vi "AutoBurn - BCU.vi"() -> ()   [LabVIEW 2013]
uses:
  <vilib>/Utility/config.llb/Write Key (String).vi
  <vilib>/Utility/config.llb/Read Key (String).vi
  <vilib>/Utility/file.llb/Read From Spreadsheet File (string).vi
  Settings/ControlCAN.dll
  <vilib>/Utility/config.llb/NI_LVConfig.lvlib
panel:
  out "?":bool
  in  "波特率 2":T1(ring)=enum."500Kbps"
  in  "错误输入（无错误）":errorcluster
  out "开始下载数据":u32
  out "开始下载数据":bool=TRUE
  out "耗时：":u32
  out "start":u32
  out "update flag":bool=TRUE
  in  "目标板类型":enum16{"BCU/主板", "BMU/从板"}(ring)
  out "Random":u32
  out "CRC16":u16 format="%x"
  out "进入烧录":bool
  out "boot模式应答计数":i32
  out "boot模式应答...成功":bool=TRUE
  out "总行数":i32
  in  "错误输入（无错误） 7":errorcluster caption="错误输入（无错误）"
  out "错误输出 18":errorcluster caption="错误输出"
  out "当前发送行":i32
  in  "错误输入（无错误） 6":errorcluster caption="错误输入（无错误）"
  out "错误输出 17":errorcluster caption="错误输出"
  in  "错误输入（无错误） 5":errorcluster caption="错误输入（无错误）"
  out "错误输出 16":errorcluster caption="错误输出"
  in  "错误输入（无错误） 4":errorcluster caption="错误输入（无错误）"
  out "错误输出 15":errorcluster caption="错误输出"
  in  "错误输入（无错误） 3":errorcluster caption="错误输入（无错误）"
  out "错误输出 14":errorcluster caption="错误输出"
  out "错误输出 13":errorcluster caption="错误输出"
  out "错误输出 12":errorcluster caption="错误输出"
  out "总电压":dbl
  out "Life":dbl
  out "返回类型":u32 format="%x"
  out "Info：":string
  in  "手动进入编程模式 2":bool
  out "T9":bool=TRUE
  out "T8":u8
  out "T7":bool=TRUE
  out "T6":bool=TRUE
  out "T5":bool=TRUE
  out "T4":bool=TRUE
  out "T3":bool=TRUE
  out "T2":bool=TRUE
  out "T1":bool=TRUE
  out "ID":u32 format="%x"
  out "错误输出 3":errorcluster caption="错误输出"
  in  "Monitor":bool
  out "校验":bool
  in  "请选择板号":u16(ring)=1 items=["BMU1"=1, "BMU2"=2, "BMU3"=3, "BMU4"=4, "BMU5"=5, "BMU6"=6, "BMU7"=7, "BMU8"=8, "BMU9"=9, "BMU10"=10, "BMU11"=11, "BMU12"=12, "BMU13"=13, "BMU14"=14, "BMU15"=15, "BMU16"=16, "BMU17"=17, "BMU18"=18, "BMU19"=19, "BMU20"=20]
  in  "手动进入编程模式":bool
  in  "板类型":enum16{"请选择板类型", "主板", "从板", "高压板"}(ring)=enum."主板"
  out "烧录结果":bool=TRUE
  out "擦除完成":bool
  out "进入烧录模式":bool
  out "MD5校验":bool
  out "进度":u8(slide) scale=0.0..100.0
  out "校验码实际值":string
  in  "校验码期望值":string
  in  "应用程序路径":path
  out "连接状态":bool=TRUE
  in  "类型":u32(ring)=4 items=["PCI5121"=1, "PCI9810"=2, "USBCAN1"=3, "USBCAN2"=4, "PCI9820"=5, "CAN232"=6, "PCI5110"=7, "CANLite(mini)"=8, "ISA9620"=9, "ISA5420"=10, "PC104CAN"=11, "CANET"=17, "DNP9810"=13, "USBCAN-E-U"=20, "USBCAN-2E-U"=21]
  in  "CAN路数":u32(ring) items=["0", "1"]
  in  "滤波方式":u8(ring) items=["Dual Filter", "Single Filter"]
  in  "工作方式":u8(ring) items=["Normal", "Listen Only"]
  in  "波特率":T1(ring)=enum."500Kbps"
  in  "设备索引":u32(ring) items=["0", "1", "2", "3", "4", "5", "6", "7", "8", "9", "10", "11", "12", "13", "14", "15", ""]
  in  "开始监控":bool
  out "CAN数据":bool
  out "Monitor_flag":bool
  out "PC端-协议类型 2":enum16{"TCP服务器Server", "TCP客户端Client"}(ring)
  out "通信端口:":u32
  out "CANET地址格式如：192.168.0.178":string
  out "发送数据长度":dbl
  out "发送的数据":i32[](array[numeric])
  in  "设备索引 4":u16(ring) items=["0", "1", "2", "3", "4", "5", "6", "7", "8", "9", "10", "11", "12", "13", "14", "15", ""]
  in  "CAN路数 4":u16(ring) items=["0", "1"]
  in  "设备类型 4":u16(ring)=4 items=["PCI5121"=1, "PCI9810"=2, "USBCAN1"=3, "USBCAN2"=4, "PCI9820"=5, "CAN232"=6, "PCI5110"=7, "CANLite(mini)"=8, "ISA9620"=9, "ISA5420"=10, "PC104CAN"=11, "CANETE"=12, "DNP9810"=13]
  out "Mode":bool
  in  "开始监控 2":bool
  out "大小":i32=426
  out "地址长度 2":u32=4
  out "数据长度 2":u32=64
  out "子字符串 2":string="9B2F9B349B399B3E9B439B499B4F9B559B5B9B619B679B6D9B739B799B7F7C7B"
  out "数据长度":u32=64
  out "地址长度":u32=4
  in  "设定":bool
  out "VCI_CAN_OBJ_T":T2 {"ID" format="%x"}
  out "子数组":string[](array[string])
  in  "从板号":dbl
  out "从板号2":dbl
  in  "读取":bool
  in  "停止 3":bool
  out "TEMP":bool
  out "CAN状态 2":bool
  out "VCI_CAN_OBJ_R":T2={"ID"=0, "TimeStamp"=0, "TimeFlag"=0, "SendType"=1, "RemoteFlag"=0, "ExternFlag"=0, "DataLen"=8, 0, 0, 0, 0, 0, 0, 0, 0, 0, 0, 0}
  in  "停止 2":bool
  out "接收":T2={"ID"=0, "TimeStamp"=61537964, "TimeFlag"=1, "SendType"=250, "RemoteFlag"=0, "ExternFlag"=0, "DataLen"=1, 255, 0, 0, 0, 0, 0, 0, 0, 0, 0, 124} {"ID" min=2 max=104373490 step=1 format="%x"; "TimeStamp" min=1962977793 max=3175728; "TimeFlag" min=1 max=0; "SendType" max=131 step=11; "RemoteFlag" min=52 max=6 step=1; "ExternFlag" max=0; "DataLen" min=1 max=170; "?" min=117 max=48 step=117; "?" min=48 max=0; "?" max=0; "?" min=2 max=0; "?" max=150 step=11; "?" min=52 max=6 step=1; "?" max=0; "?" min=1 max=170; "?" min=120 max=175; "?" max=12; "?" max=0}
  out "收到请求":bool=TRUE
  out "分配":bool
  out "设置中？ 2":bool
  in  "Boar_Type":bool
  out "temp1":bool
  out "设置中？":bool
  in  "总步骤":dbl=21.0
  in  "失败重测次数":dbl=3.0
  out "一键测试":bool
  out "测试结果":bool
  in  "行号":dbl=21.0
  in  "工作方式 2":u8(ring) items=["Normal", "Listen Only"]
  in  "设备类型 2":u16(ring)=4 items=["PCI5121"=1, "PCI9810"=2, "USBCAN1"=3, "USBCAN2"=4, "PCI9820"=5, "CAN232"=6, "PCI5110"=7, "CANLite(mini)"=8, "ISA9620"=9, "ISA5420"=10, "PC104CAN"=11, "CANETE"=12, "DNP9810"=13]
  in  "停止":bool
  out "CAN状态":bool=TRUE
  in  "监控":bool
  # "当前BMU信息"
  # "蓝微新源BMS_CAN应用程序下载器V1.0.7D"
  # "注意：升级完成后系统需要重新上电才能正常运行！"
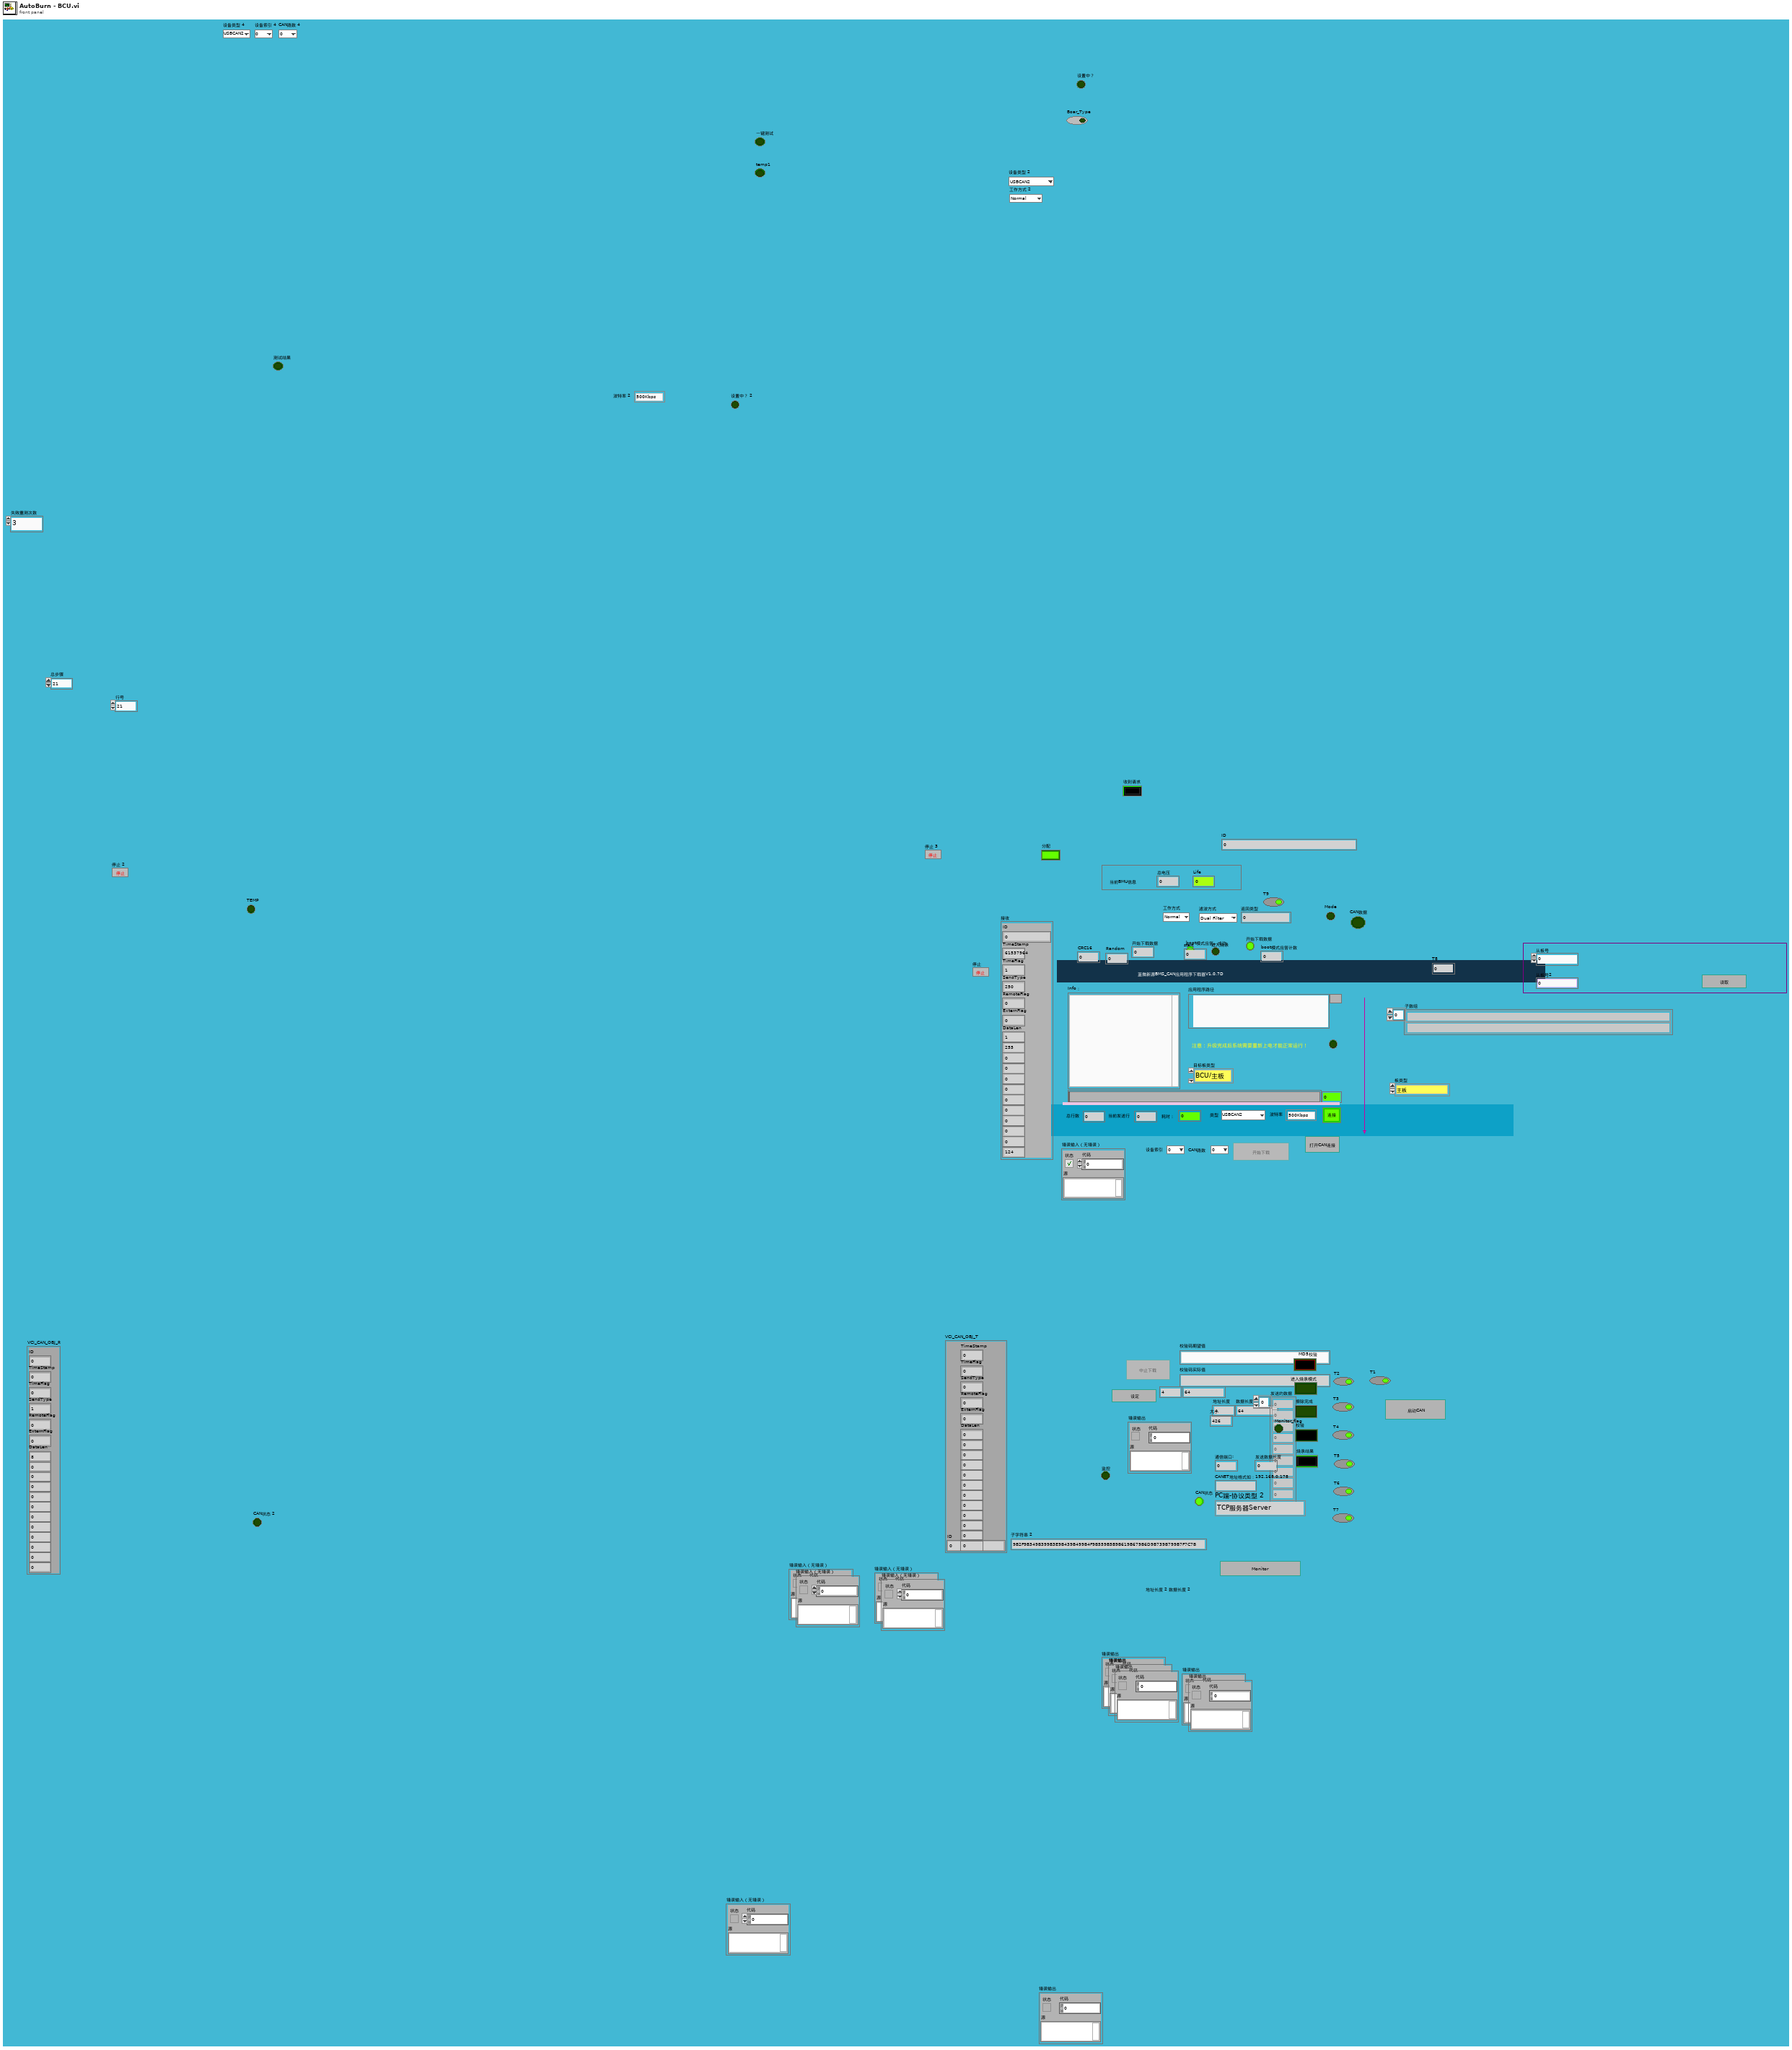
[diagram p1: front panel]
types:
  T1 = enum16{"5Kbps", "10Kbps", "20Kbps", "40Kbps", "50Kbps", "80Kbps", "100Kbps", "125Kbps", "200Kbps", "250Kbps", "400Kbps", "500Kbps", "666Kbps", "800Kbps", "1000Kbps"}
  T2 = cluster{"ID":u32, "TimeStamp":u32, "TimeFlag":u8, "SendType":u8, "RemoteFlag":u8, "ExternFlag":u8, "DataLen":u8, u8, u8, u8, u8, u8, u8, u8, u8, u8, u8, u8}
  T3 = enum8{"Enabled", "Disabled", "Disabled and Grayed Out"}
  T4 = typedef "NI_LVConfig.lvlib/Config Data RefNum.ctl" = refnum<k1>
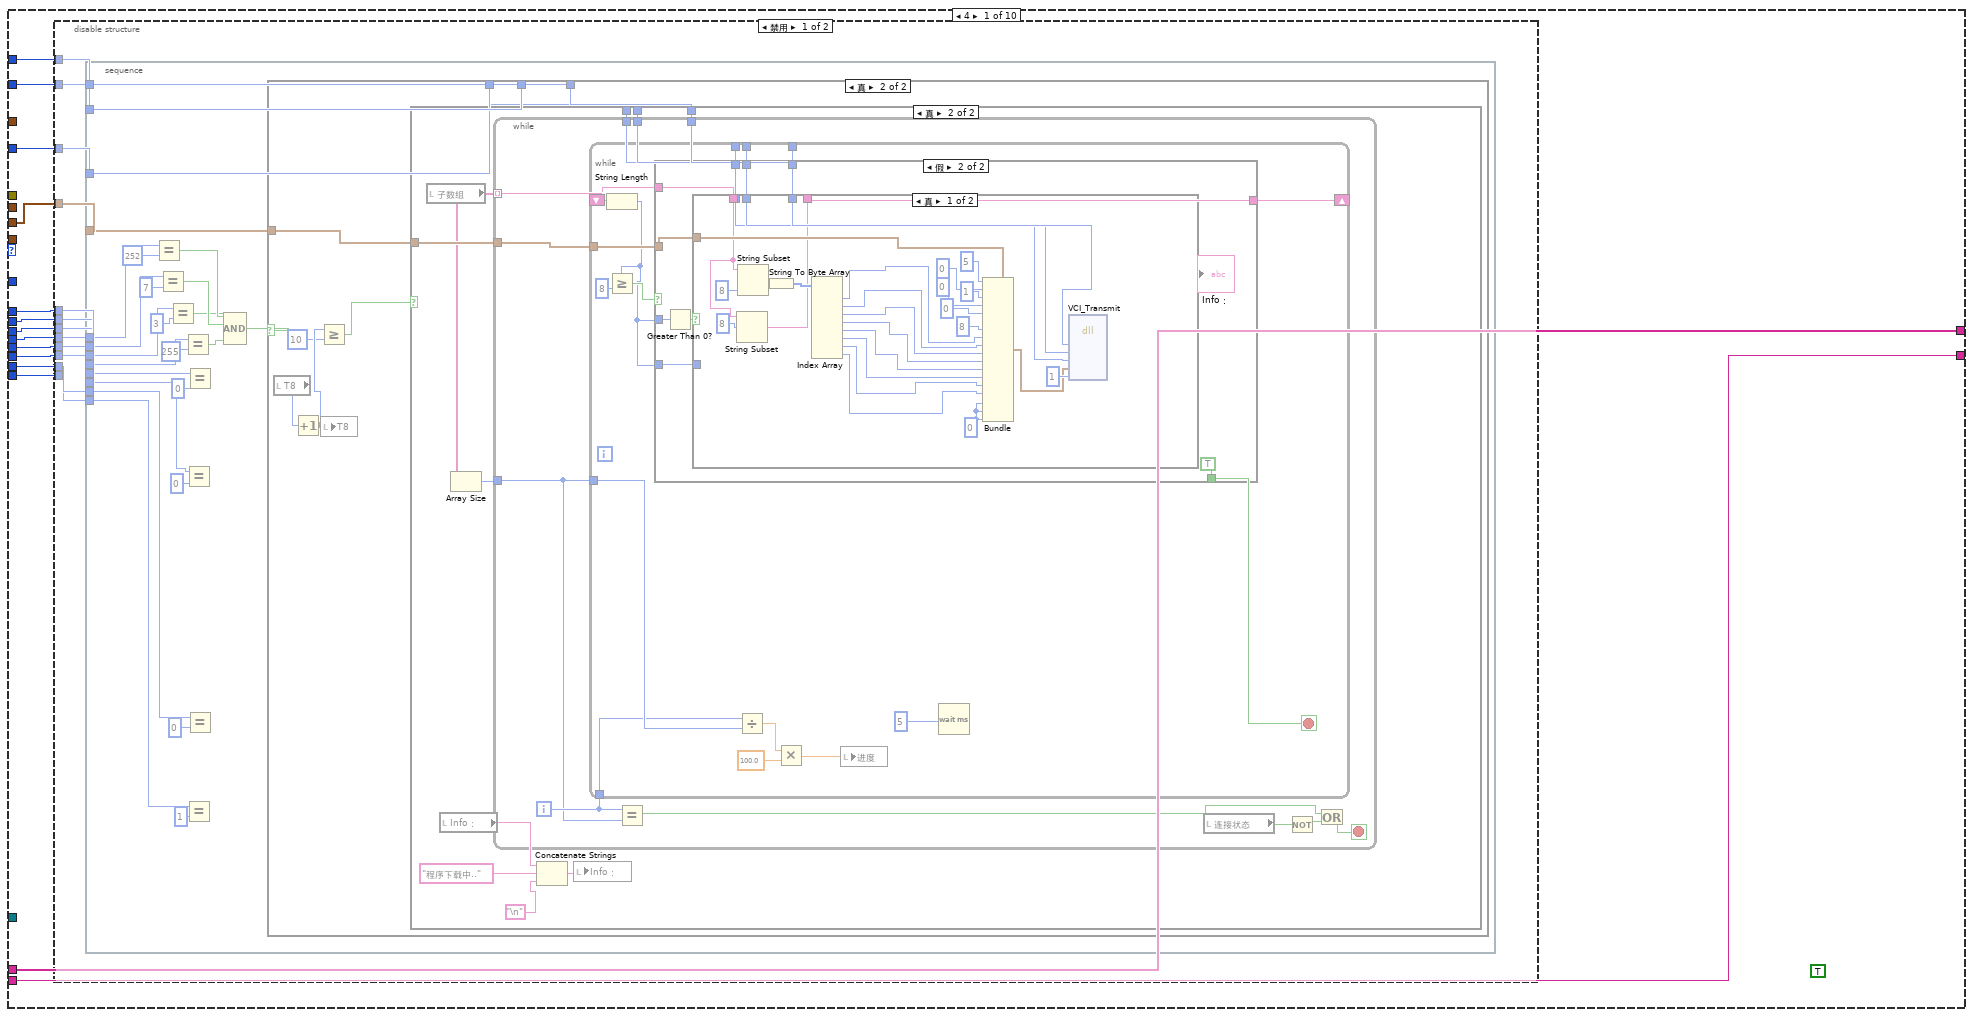
[diagram p3: hidden frame]
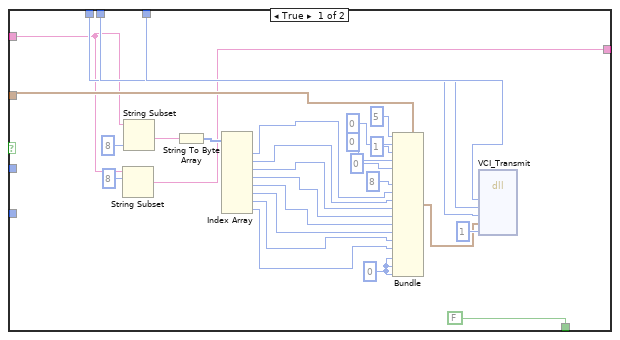
[diagram p6: hidden frame]
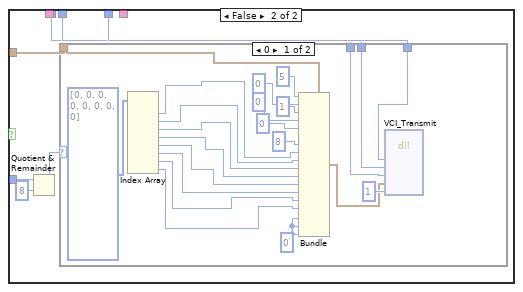
[diagram p7: hidden frame]
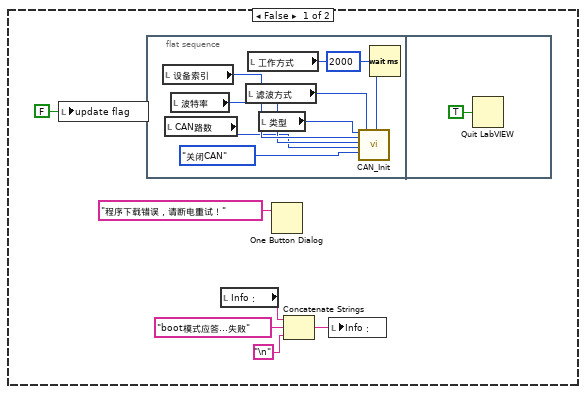
[diagram p10: hidden frame]
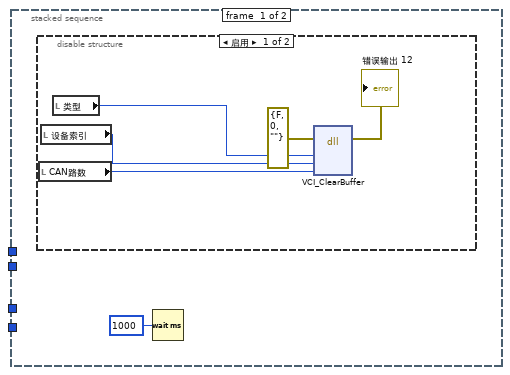
[diagram p11: hidden frame]
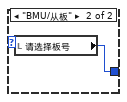
[diagram p13: hidden frame]
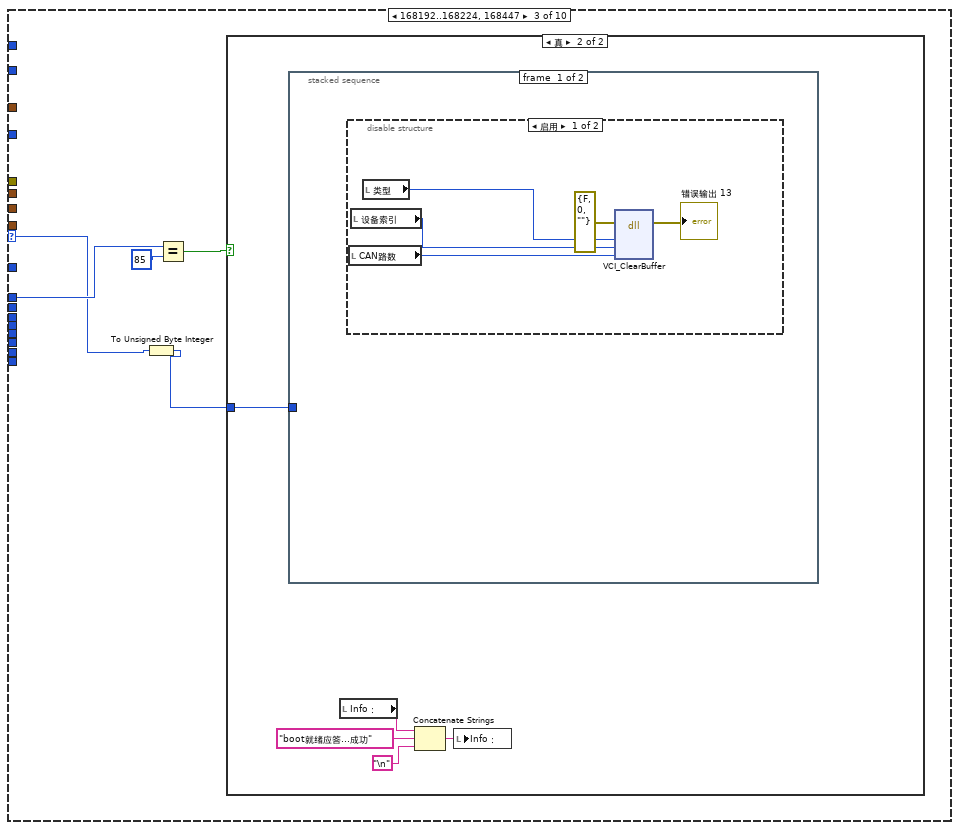
[diagram p14: hidden frame]
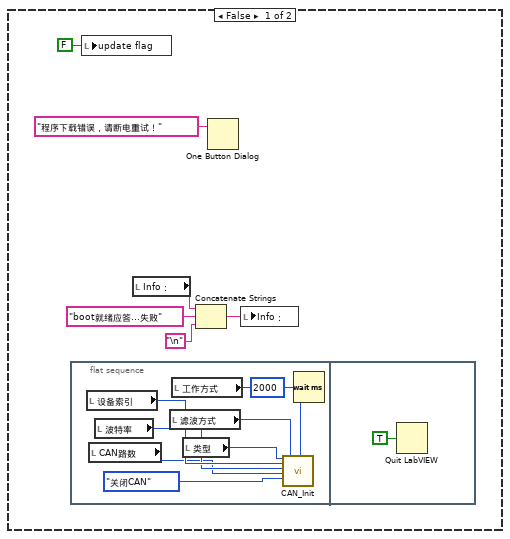
[diagram p15: hidden frame]
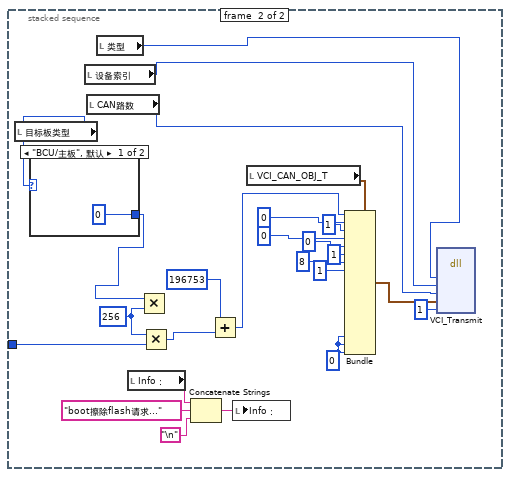
[diagram p17: hidden frame]
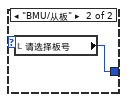
[diagram p18: hidden frame]
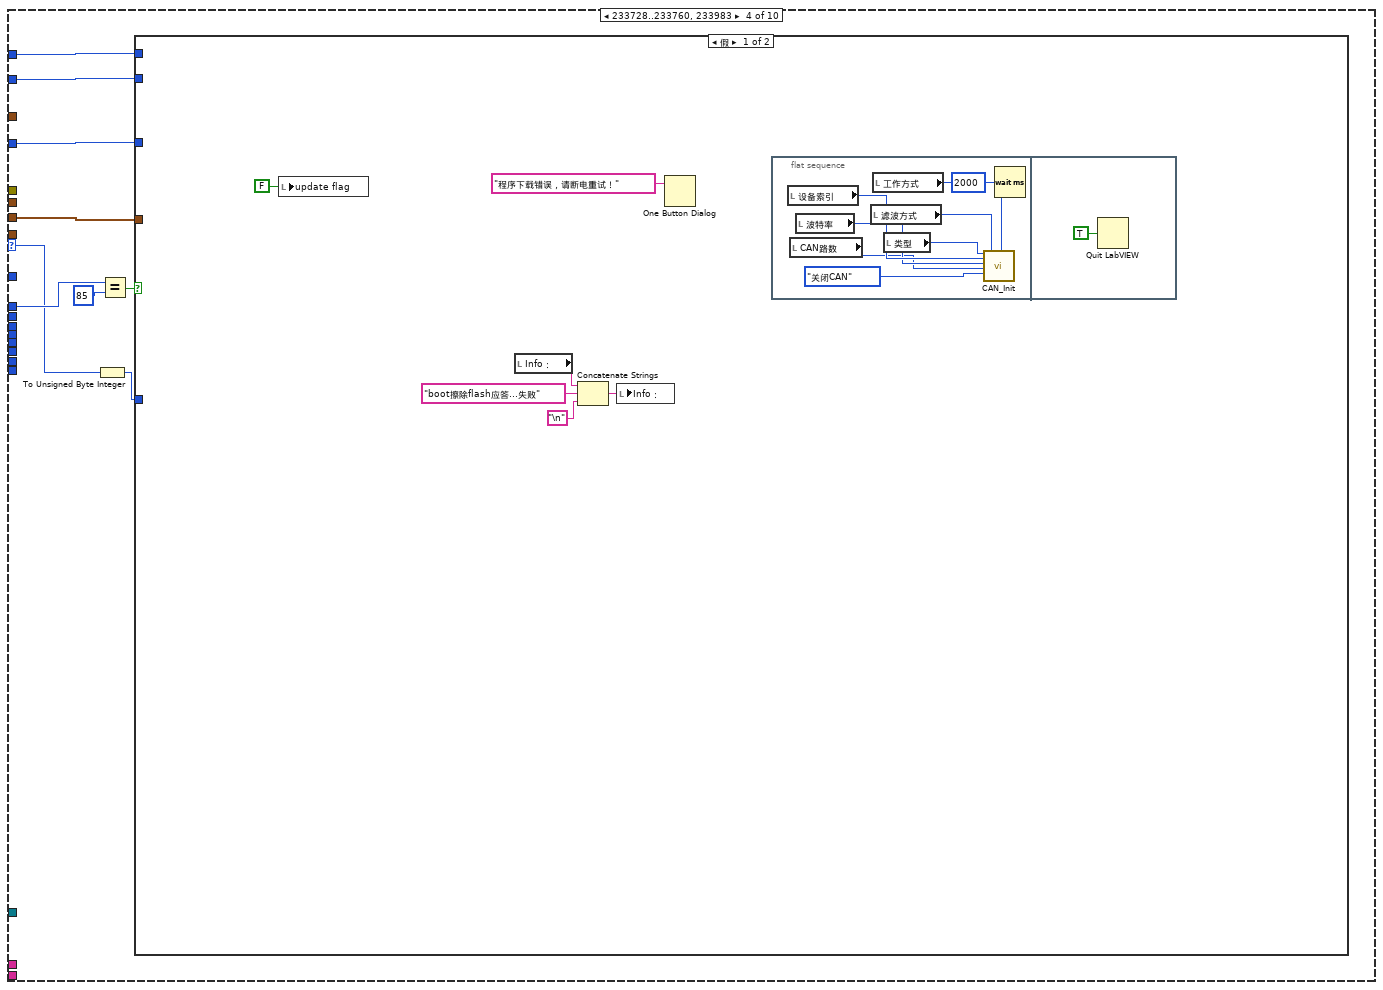
[diagram p19: hidden frame]
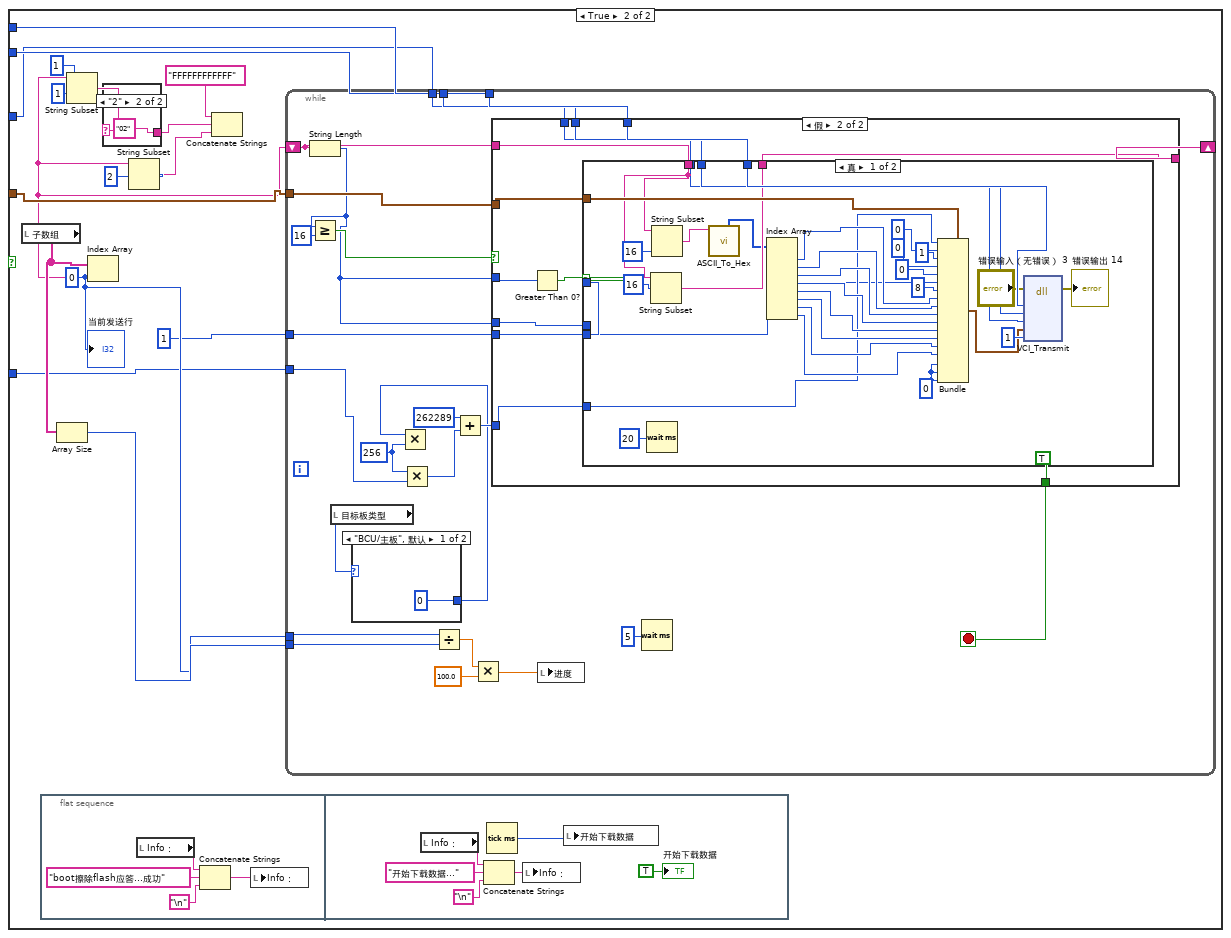
[diagram p20: hidden frame]
diagram:
  (unwired) u32 0
  (unwired) u32 255
  w21 = "" ("布尔文本.文本")
  w22 = cluster{u32, u32}[] [{0, 0}] ("颜色[4]")
  w29 = "" ("校验码期望值")
  w37 = FALSE ("进入烧录模式")
  n1 = local write "TEMP"(FALSE ("TEMP")) -> ()
  n2 = local read "VCI_CAN_OBJ_R"() -> (w19:T2)
  n3 = local write "校验码期望值"(w29) -> ()
  n4 = local write "校验码实际值"(w29) -> ()
  n5 = property on="校验" class="Bool (严格)"("Colors [4]"=w22, "BoolText.Text"=w21) -> ()  [unwired: 2 in, 2 out]
  n6 = Obtain Queue(name (unnamed)="CAN1" ("名称（未命名）"), element data type=w19, error in (no error)="错误输入（无错误）") -> (queue out=w20:refnum<queue>, error out=w7:errorcluster)  [unwired: 2 in, 1 out]
  n7 = property on="烧录结果" class="Bool (严格)"("Colors [4]"=w22, "BoolText.Text"=w21) -> ()  [unwired: 2 in, 2 out]
  n8 = Initialize Array("", 1 ("维数大小")) -> (w33:string[])
  n9 = local write "连接状态"(FALSE ("连接状态")) -> ()
  n10 = local write "boot模式应答...成功"(FALSE ("boot模式应答...成功")) -> ()
  n11 = local write "开始下载数据"(u32 0 ("开始下载数据")) -> ()
  n12 = local write "耗时："(u32 0 ("耗时：")) -> ()
  n13 = property on="请选择板号" class="Ring (严格)"("Visible"=TRUE ("可见")) -> ()  [unwired: 2 in, 2 out]
  n14 = local write "耗时："(u32 0 ("耗时：")) -> ()
  n15 = stacked-sequence {
    tunnel: "错误输入（无错误）" -> [w57 w89 w200]
    tunnel: [w52 _ _] -> w1
    frame #0 {
      w83 = "BURNRESULT" ("section")
      w87 = u32 21 items=["PCI5121"=1, "PCI9810"=2, "USBCAN1"=3, "USBCAN2"=4, "PCI9820"=5, "CAN232"=6, "PCI5110"=7, "CANLite(mini)"=8, "ISA9620"=9, "ISA5420"=10, "PC104CAN"=11, "CANET"=17, "DNP9810"=13, "USBCAN-E-U"=20, "USBCAN-2E-U"=21] ("类型")
      w86 = u32 4 items=["PCI5121"=1, "PCI9810"=2, "USBCAN1"=3, "USBCAN2"=4, "PCI9820"=5, "CAN232"=6, "PCI5110"=7, "CANLite(mini)"=8, "ISA9620"=9, "ISA5420"=10, "PC104CAN"=11, "CANET"=17, "DNP9810"=13, "USBCAN-E-U"=20, "USBCAN-2E-U"=21] ("类型")
      # "识别CAN卡，文件路径等"
      n16 = call <vilib>:"Open Config Data.vi"("error in (no error)"=w57, "configuration file path"=path "D:/BlueWay/configresult.ini") -> ("error out"=w81:errorcluster, "refnum"=w84:T4)  [unwired: 7 in, 1 out]
      n17 = call <vilib>:"Open Config Data.vi"("error in (no error)"=w57, "configuration file path"=path "D:/BlueWay/BMU从板号.ini") -> ("error out"=w67:errorcluster, "refnum"=w65:T4)  [unwired: 7 in, 1 out]
      n18 = call <vilib>:"Open Config Data.vi"("error in (no error)"=w57, "configuration file path"=path "D:/自动测试项目文件/ProjectSetting.ini") -> ("error out"=w72:errorcluster, "refnum"=w71:T4)  [unwired: 7 in, 1 out]
      n19 = call-poly <vilib>:"Write Key.vi"("section"=w83, "error in (no error)"=w81, "value"="FAIL" ("section"), "key"=w83, "refnum"=w84) -> ("error out"=w79:errorcluster, "refnum out"=w80:T4)  [unwired: 4 in, 1 out]
      n20 = call <vilib>:"Close Config Data.vi"("error in (no error)"=w79, "refnum"=w80) -> ()  [unwired: 8 in, 2 out]
      n21 = Select(t=w86, s=TRUE, f=w87) -> (s? t:f=w88:u32)
      n22 = call-poly <vilib>:"Read Key.vi"("section"="BMUNO", "error in (no error)"=w67, "key"="BMUNO", "refnum"=w65) -> ("error out"=w48:errorcluster, "value"=w73:string, "refnum out"=w49:T4)  [unwired: 4 in, 1 out]
      n23 = local write "类型"(w88) -> ()
      n24 = Decimal String To Number(string=w73) -> (number=w56:i32)  [unwired: 2 in, 1 out]
      n25 = local write "请选择板号"(w56) -> ()
      n26 = call-poly <vilib>:"Read Key.vi"("section"="PROJECT", "error in (no error)"=w72, "key"="内部CAN波特率", "refnum"=w71) -> ("error out"=w53:errorcluster, "value"=w70:string, "refnum out"=w75:T4)  [unwired: 4 in, 1 out]
      n27 = call-poly <vilib>:"Read Key.vi"("section"="PROJECT", "error in (no error)"=w53, "key"="BCU应用程序" ("字符串"), "refnum"=w75) -> ("error out"=w52:errorcluster, "value"=w76:string)  [unwired: 4 in, 2 out]
      n28 = call-poly <vilib>:"Read Key.vi"("section"="BCUTYPE", "error in (no error)"=w48, "key"="BCUTYPE", "refnum"=w49) -> ("error out"=w46:errorcluster, "value"=w44:string, "refnum out"=w47:T4)  [unwired: 4 in, 1 out]
      n29 = Equal?(x=w70, y="500K") -> (x = y?=w61:bool)
      n30 = Select(t=T1."500Kbps" ("波特率"), s=w61, f=T1."250Kbps" ("波特率")) -> (s? t:f=w55:T1)
      n31 = Build Path(base path=path "D:/自动测试项目文件" ("基路径"), name or relative path=w76) -> (appended path=w42:path)
      n32 = local write "波特率"(w55) -> ()
      n33 = Equal?(x=w44, y="通用") -> (x = y?=w45:bool)
      n34 = call <vilib>:"Close Config Data.vi"("error in (no error)"=w46, "refnum"=w47) -> ()  [unwired: 8 in, 2 out]
      n35 = Select(t=path "D:/BlueWay/通用文件/TYXXXXMSXXXX.s19" ("基路径"), s=w45, f=w42) -> (s? t:f=w40:path)
      n36 = local write "应用程序路径"(w40) -> ()
    }
    frame #1 {
      n37 = local read "应用程序路径"() -> (w90:path)
      n38 = Not A Number/Path/Refnum?(number/path/refnum=w90) -> (NaN/Path/Refnum?=w94:bool)
      n39 = Strip Path(path=w90) -> (name=w97:string)  [unwired: 1 out]
      n40 = String Subset(string=w97, offset (0)=6 ("偏移量(0)"), length (rest)=2 ("长度（剩余）")) -> (substring=w93:string)
      n41 = case shown="\"MS\"" w93 {
        tunnel: [TRUE ("y") FALSE ("y") FALSE ("y")] -> w96
        frame "假", Default {
          n42 = local read "Info："() -> (w99:string)
          n43 = Concatenate Strings(w99, "无法识别板类型！\n" ("字符串")) -> (w101:string)
          n44 = local write "Info："(w101) -> ()
        }
        frame "MS" {
          n45 = local read "Info："() -> (w103:string)
          n46 = local write "目标板类型"(enum16{"BCU/主板", "BMU/从板"}."BCU/主板" ("类型")) -> ()
          n47 = property on="请选择板号" class="Ring (严格)"("Visible"=FALSE ("可见")) -> ()  [unwired: 2 in, 2 out]
          n48 = Concatenate Strings(w103, "通过文件识别为主板！\n" ("字符串")) -> (w104:string)
          n49 = local write "Info："(w104) -> ()
        }
        frame "SS" {
          n50 = local read "Info："() -> (w109:string)
          n51 = local write "目标板类型"(enum16{"BCU/主板", "BMU/从板"}."BMU/从板" ("类型")) -> ()
          n52 = property on="请选择板号" class="Ring (严格)"("Visible"=TRUE ("可见")) -> ()  [unwired: 2 in, 2 out]
          n53 = Concatenate Strings(w109, "通过文件识别为从板！\n" ("字符串")) -> (w110:string)
          n54 = local write "Info："(w110) -> ()
        }
      }
      n55 = Or(x=w94, y=w96) -> (x .or. y?=w95:bool)
      n56 = case shown="假" w95 {
        tunnel: w90 -> [w150 _]
        tunnel: w89 -> [w114 _]
        frame False {
          n57 = Path To String(path=w150) -> (string=w125:string)
          n58 = local read "Info："() -> (w121:string)
          n59 = String Subset(string=w125, offset (0)=6 ("偏移量(0)"), length (rest)=2 ("长度（剩余）")) -> (substring=w122:string)
          n60 = call-poly <vilib>:"Read From Spreadsheet File.vi"("file path (dialog if empty)"=w150) -> ("all rows"=w152:string[][])  [unwired: 6 in, 4 out]
          n61 = call <vilib>:"Space Constant.vi"() -> ("String"=w148:string)
          n62 = Search and Replace String(replace all?=TRUE ("替换全部？(F)"), input string=w125, search string=w148, replace string="" ("替换字符串(\"\")")) -> (result string=w135:string)  [unwired: 4 in, 3 out]
          n63 = case shown="\"真\"" w122 {
            frame "假", Default {
            }
            frame "真" {
            }
          }
          n64 = Concatenate Strings(w121, "文件加载成功！\n" ("字符串")) -> (w119:string)
          n65 = Index Array(array=w152, index (col)=0 ("禁用的索引 (列)")) -> (element=w139:string[])  [unwired: 1 in]
          n66 = Search/Split String(string=w135, search string/char (-)="(MD5=" ("搜索字符串/字符(-)")) -> (match + rest of string=w132:string, offset of match=w142:i32)  [unwired: 1 in, 1 out]
          n67 = local write "Info："(w119) -> ()
          n68 = Delete From Array(array=w139, length=1 ("长度"), index=0 ("索引")) -> (array with subset deleted=w131:string[])  [unwired: 1 out]
          n69 = call <vilib>:"MD5Checksum File.vi"("error in (no error)"=w114, "Path"=w150) -> ("MD5 message-digest"=w116:string)  [unwired: 8 in, 1 out]
          n70 = Array Size(array=w131) -> (size(s)=w129:i32)
          n71 = Decrement(x=w129) -> (x-1=w128:i32)
          n72 = Delete From Array(array=w131, length=1 ("长度"), index=w128) -> (array with subset deleted=w127:string[])  [unwired: 1 out]
          n73 = Array Size(array=w127) -> (size(s)=w115:i32)
          n74 = local write "校验码实际值"(w116) -> ()
          n75 = Add(x=w142, y=5) -> (x+y=w143:i32)
          n76 = Search/Split String(string=w135, search string/char (-)=")" ("搜索字符串/字符(-)")) -> ()  [unwired: 1 in, 3 out]
          n77 = String Subset(string=w132, offset (0)=45 ("偏移量(0)"), length (rest)=8 ("长度（剩余）")) -> ()  [unwired: 1 out]
          n78 = local write "总行数"(w115) -> ()
          n79 = String Subset(string=w135, offset (0)=w143, length (rest)=32 ("长度（剩余）")) -> (substring=w133:string)
          n80 = Equal?(x=w133, y=w116) -> (x = y?=w140:bool)
          n81 = case shown="真" w140 {
            frame False {
              n82 = Build Array(cluster{u32, u32} {16711680, 0}) -> (w182:cluster{u32, u32}[])
              n83 = property on="MD5校验" class="Bool (严格)"("Colors [4]"=w182, "BoolText.Text"="失败" ("布尔文本.文本")) -> ()  [unwired: 2 in, 2 out]
            }
            frame True {
              n84 = Build Array(cluster{u32, u32} {6618880, 0}) -> (w185:cluster{u32, u32}[])
              n85 = property on="MD5校验" class="Bool (严格)"("Colors [4]"=w185, "BoolText.Text"="成功" ("布尔文本.文本")) -> ()  [unwired: 2 in, 2 out]
            }
          }
          n86 = local write "校验码期望值"(w133) -> ()
          n87 = for {
            tunnel: w127 -> [w163] mode=indexing
            shift-right: [w161] -> w117
            shift-left: u16 0 ("偏移量(0)") -> [w162]
            tunnel: [w155] -> w118 mode=indexing
            n88 = String Subset(string=w163, offset (0)=1 ("偏移量(0)"), length (rest)=1 ("长度（子字符串长度）")) -> (substring=w166:string)
            n89 = case shown="\"1\", 默认" w166 {
              tunnel: ["01" ("子字符串(\"\")") "02" ("子字符串(\"\")")] -> w167
              frame "1", Default {
              }
              frame "2" {
              }
            }
            n90 = String Subset(string=w163, offset (0)=2 ("偏移量(0)")) -> (substring=w169:string)  [unwired: 1 in]
            n91 = Concatenate Strings("FFFFFFFFFFFF" ("子字符串(\"\")"), w167, w169) -> (w155:string)
            n92 = String Subset(string=w155, offset (0)=12 ("偏移量(0)")) -> (substring=w153:string)  [unwired: 1 in]
            n93 = String Length(string=w153) -> (length=w160:i32)
            n94 = Divide(x=w160, y=2) -> (x/y=w158:dbl)
            n95 = for {
              N: w158 -> [_]
              tunnel: w153 -> [w178]
              shift-right: [w173] -> w156
              shift-left: u16 0 ("偏移量(0)") -> [w171]
              i -> [w177]
              w175 = 2 ("x")
              n96 = Multiply(x=w175, y=w177) -> (x*y=w176:i32)
              n97 = String Subset(string=w178, offset (0)=w176, length (rest)=w175) -> (substring=w174:string)
              n98 = call "ASCII_To_Hex.vi"("ASCII String"=w174) -> ("hex1"=w172:u8)  [unwired: 6 in, 4 out]
              n99 = Add(x=w171, y=w172) -> (x+y=w173:u16)
            }
            n100 = Add(x=w162, y=w156) -> (x+y=w161:u16)
          }
          n101 = local write "CRC16"(w117) -> ()
          n102 = local write "子数组"(w118) -> ()
        }
        frame True {
          n103 = flat-sequence {
            frame #0 {
              n104 = local read "Info："() -> (w188:string)
              n105 = Concatenate Strings(w188, "文件加载错误！\n" ("字符串")) -> (w187:string)
              n106 = local write "Info："(w187) -> ()
            }
            frame #1 {
              n107 = Wait (ms)(milliseconds to wait=u32 2000 ("等待时间（毫秒）")) -> ()  [unwired: 1 out]
            }
            frame #2 {
              n108 = local read "设备索引"() -> (w192:u32)
              n109 = local read "CAN路数"() -> (w194:u32)
              n110 = local read "波特率"() -> (w193:T1)
              n111 = local read "滤波方式"() -> (w195:u8)
              n112 = local read "工作方式"() -> (w196:u8)
              n113 = local read "类型"() -> (w191:u32)
              n114 = call "CAN_Init.vi"("设备类型"=w191, "设备索引"=w192, "波特率"=w193, "CAN路数"=w194, "操作类型"=enum16{"初始化CAN", "关闭CAN"}."关闭CAN", "滤波方式"=w195, "工作方式"=w196) -> ()  [unwired: 11 in, 2 out]
            }
            frame #3 {
              n115 = Quit LabVIEW(quit? (T)=TRUE ("退出？(T)")) -> ()
            }
          }
        }
      }
    }
    frame #2 {
      w204 = "" ("布尔文本.文本")
      w205 = cluster{u32, u32}[] [{0, 0}] ("颜色[4]")
      w206 = FALSE
      n116 = local write "update flag"(TRUE ("update flag")) -> ()
      n117 = property on="烧录结果" class="Bool (严格)"("Colors [4]"=w205, "BoolText.Text"=w204) -> ()  [unwired: 2 in, 2 out]
      n118 = local read "设备索引"() -> (w213:u32)
      n119 = local read "CAN路数"() -> (w211:u32)
      n120 = local read "波特率"() -> (w212:T1)
      n121 = local read "滤波方式"() -> (w210:u8)
      n122 = local read "工作方式"() -> (w209:u8)
      n123 = local read "类型"() -> (w214:u32)
      n124 = property on="校验" class="Bool (严格)"("Colors [4]"=w205, "BoolText.Text"=w204) -> ()  [unwired: 2 in, 2 out]
      n125 = call "CAN_Init.vi"("设备类型"=w214, "设备索引"=w213, "波特率"=w212, "CAN路数"=w211, "操作类型"=enum16{"初始化CAN", "关闭CAN"}."初始化CAN", "error in (no error)"=w200, "滤波方式"=w210, "工作方式"=w209) -> ("CAN 操作结果"=w202:bool, "error out"=w199:errorcluster)  [unwired: 10 in]
      n126 = local write "擦除完成"(w206) -> ()
      n127 = local write "进度"(u8 0 ("进度")) -> ()
      n128 = local write "进入烧录模式"(w206) -> ()
      n129 = local write "烧录结果"(w206) -> ()
      n130 = local write "Monitor_flag"(FALSE ("Monitor_flag")) -> ()
      n131 = local write "CAN状态"(w202) -> ()
      n132 = local write "连接状态"(w202) -> ()
      n133 = case shown="真" w202 {
        tunnel: w200 -> [w215 _]
        tunnel: w199 -> [_ _]
        frame True {
          n134 = local read "Info："() -> (w216:string)
          n135 = stacked-sequence {
            tunnel: w215 -> [w224 _ _]
            tunnel: [w223 _ _] -> _
            frame #0 {
              n136 = disable-structure shown="启用" {
                disable-tunnel: w224 -> [w227 _]
                disable-tunnel: [w226 _] -> w223
                frame Enabled {
                  n137 = local read "CAN路数"() -> (w228:u32)
                  n138 = local read "设备索引"() -> (w229:u32)
                  n139 = local read "类型"() -> (w230:u32)
                  n140 = dll-call lib="F:/Bluewave New Energy/SVN_Work/BMS_BootLoader/trunk/BMS_Bootloader/AutoBurn/Settings/ControlCAN.dll" fn="VCI_ClearBuffer" label="VCI_Clearbuffer"(error in=w227, "DeviceType"=w230, "DeviceInd"=w229, "CANInd"=w228) -> (error out=w226:errorcluster)  [unwired: 3 in, 4 out]
                }
                frame Disabled {
                }
              }
              n141 = local write "boot模式应答...成功"(FALSE) -> ()
              n142 = local write "开始下载数据"(FALSE ("开始下载数据")) -> ()
              n143 = local write "进入烧录"(TRUE ("布尔")) -> ()
              n144 = local write "开始下载数据"(u32 0 ("开始下载数据")) -> ()
            }
            frame #1 {
              w236 = TRUE ("T1")
              w235 = TRUE ("T1")
              n145 = local read "Info："() -> (w231:string)
              n146 = Concatenate Strings(w231, "boot模式请求..." ("字符串"), "\n") -> (w234:string)
              n147 = local write "Info："(w234) -> ()
              n148 = local write "T2"(w235) -> ()
              n149 = local write "T3"(w236) -> ()
              n150 = local write "T1"(w235) -> ()
              n151 = local write "T4"(w236) -> ()
              n152 = local write "T5"(w236) -> ()
              n153 = local write "T6"(w236) -> ()
              n154 = local write "T7"(w236) -> ()
              n155 = local write "T8"(u8 0 ("T8")) -> ()
              n156 = local write "T9"(w236) -> ()
            }
            frame #2 {
              n157 = local read "目标板类型"() -> (w240:enum16{"BCU/主板", "BMU/从板"})
              n158 = case shown="\"BCU/主板\", 默认" w240 {
                tunnel: [u16 0 ("请选择板号") w253] -> w241
                frame "BCU/主板", Default {
                }
                frame "BMU/从板" {
                  n159 = local read "请选择板号"() -> (w253:u16)
                }
              }
              n160 = Tick Count (ms)() -> (millisecond timer value=w239:u32)
              n161 = local write "start"(w239) -> ()
              n162 = local write "boot模式应答计数"(0 ("boot模式应答计数")) -> ()
              n163 = Multiply(x=w241, y=u16 256) -> (x*y=w244:u16)
              n164 = Add(x=u32 65681 ("ID"), y=w244) -> (x+y=w242:u32)
              n165 = local read "VCI_CAN_OBJ_T"() -> (w246:T2)
              n166 = case shown="1, 默认" w241 {
                tunnel: [w258 w270] -> w250
                tunnel: w246 -> [w257 w269]
                tunnel: w242 -> [w255 w267]
                frame 0 {
                  w254 = u8 170
                  w261 = u8 0 ("元素")
                  n167 = Bundle(cluster=w257, "ID"=w255, "TimeStamp"=u8 0 ("RemoteFlag"), "TimeFlag"=u8 1, "SendType"=u8 0 ("DataLen"), "RemoteFlag"=u8 0, "ExternFlag"=u8 1, "DataLen"=u8 8, u8 1 ("元素"), w254, w254, w254, w254, w261, w261, w261) -> (w258:T2)  [unwired: 3 in]
                }
                frame 1, Default {
                  w266 = u8 187
                  w273 = u8 0 ("元素")
                  n168 = Bundle(cluster=w269, "ID"=w267, "TimeStamp"=u8 0 ("RemoteFlag"), "TimeFlag"=u8 1, "SendType"=u8 0 ("DataLen"), "RemoteFlag"=u8 0, "ExternFlag"=u8 1, "DataLen"=u8 8, u8 1 ("元素"), w266, w266, w266, w266, w273, w273, w273) -> (w270:T2)  [unwired: 3 in]
                }
              }
              n169 = local read "设备索引"() -> (w248:u32)
              n170 = local read "CAN路数"() -> (w247:u32)
              n171 = local read "类型"() -> (w249:u32)
              n172 = dll-call lib="F:/Bluewave New Energy/SVN_Work/BMS_BootLoader/trunk/BMS_Bootloader/AutoBurn/Settings/ControlCAN.dll" fn="VCI_Transmit"("DeviceType"=w249, "DeviceInd"=w248, "CANInd"=w247, "pSend"=w250, "Len"=u32 1) -> ()  [unwired: 5 in, 6 out]
            }
          }
          n173 = Concatenate Strings(w216, "启动CAN成功.." ("字符串"), "\n") -> (w219:string)
          n174 = local write "Info："(w219) -> ()
        }
        frame False {
          n175 = stacked-sequence {
            frame #0 {
              n176 = local read "Info："() -> (w278:string)
              n177 = Concatenate Strings(w278, "启动CAN失败.." ("字符串"), "\n") -> (w281:string)
              n178 = local write "Info："(w281) -> ()
            }
            frame #1 {
              n179 = local read "设备索引"() -> (w284:u32)
              n180 = local read "CAN路数"() -> (w286:u32)
              n181 = local read "波特率"() -> (w285:T1)
              n182 = local read "滤波方式"() -> (w287:u8)
              n183 = local read "工作方式"() -> (w288:u8)
              n184 = local read "类型"() -> (w283:u32)
              n185 = Wait (ms)(milliseconds to wait=u32 2000 ("等待时间（毫秒）")) -> ()  [unwired: 1 out]
              n186 = call "CAN_Init.vi"("设备类型"=w283, "设备索引"=w284, "波特率"=w285, "CAN路数"=w286, "操作类型"=enum16{"初始化CAN", "关闭CAN"}."关闭CAN", "滤波方式"=w287, "工作方式"=w288) -> ()  [unwired: 11 in, 2 out]
            }
            frame #2 {
              n187 = Quit LabVIEW(quit? (T)=TRUE ("退出？(T)")) -> ()
            }
          }
        }
      }
    }
  }
  n188 = while {
    tunnel: w20 -> [w296]
    tunnel: [w295] -> w3
    tunnel: w1 -> [w294]
    tunnel: [w293] -> w2
    tunnel: w19 -> [w291]
    stop <- "停止 2" stop-if-true
    n189 = local read "连接状态"() -> (w292:bool)
    n190 = case shown="真" w292 {
      tunnel: w296 -> [w304 w323]
      tunnel: [w304 w322] -> w295
      tunnel: w294 -> [w299 w321]
      tunnel: [w299 w320] -> w293
      tunnel: [w298 _] -> _
      tunnel: w291 -> [_ w308]
      frame False {
        n191 = local read "设备索引"() -> (w301:u32)
        n192 = local read "CAN路数"() -> (w300:u32)
        n193 = local read "类型"() -> (w302:u32)
        n194 = dll-call lib="F:/Bluewave New Energy/SVN_Work/BMS_BootLoader/trunk/BMS_Bootloader/AutoBurn/Settings/ControlCAN.dll" fn="VCI_ClearBuffer" label="VCI_Clearbuffer"(error in=w299, "DeviceType"=w302, "DeviceInd"=w301, "CANInd"=w300) -> (error out=w298:errorcluster)  [unwired: 3 in, 4 out]
        n195 = Wait (ms)(milliseconds to wait=u32 50 ("等待时间（毫秒）")) -> ()  [unwired: 1 out]
      }
      frame True {
        (unwired) TRUE
        n196 = local read "CAN路数"() -> (w310:u32)
        n197 = local read "设备索引"() -> (w311:u32)
        n198 = local read "类型"() -> (w312:u32)
        n199 = dll-call lib="F:/Bluewave New Energy/SVN_Work/BMS_BootLoader/trunk/BMS_Bootloader/AutoBurn/Settings/ControlCAN.dll" fn="VCI_Receive"(error in=w321, "DeviceType"=w312, "DeviceInd"=w311, "CANInd"=w310, "pReceive"=w308, "Len"=u32 1, "WaitTime"=10) -> (error out=w315:errorcluster, "返回类型"=w316:u32, "pReceive"=w314:T2)  [unwired: 7 in, 1 out]
        "接收" <- w314
        n200 = Equal?(x=w316, y=1) -> (x = y?=w305:bool)
        n201 = Unbundle(w314) -> ("ID"=w306:u32, w309:u8)  [unwired: 16 out]
        "ID" <- w306
        "返回类型" <- w306
        n202 = Equal?(x=u32 4, y=w306) -> (x = y?=w307:bool)
        n203 = And(x=w307, y=w305) -> ()  [unwired: 1 out]
        n204 = case shown="真" w305 {
          tunnel: w323 -> [w325 w336]
          tunnel: [w325 w335] -> w322
          tunnel: w314 -> [_ w334]
          tunnel: w315 -> [w324 w333]
          tunnel: [w324 w332] -> w320
          tunnel: w309 -> [_ w329]
          tunnel: w312 -> [_ w328]
          tunnel: w311 -> [_ w327]
          tunnel: w310 -> [_ w326]
          frame False {
          }
          frame True {
            n205 = disable-structure shown="禁用" {
              disable-tunnel: w329 -> [w342 _]
              disable-tunnel: w328 -> [w340 _]
              disable-tunnel: w327 -> [w339 _]
              disable-tunnel: w326 -> [w338 _]
              frame Disabled {
                n206 = Equal?(x=w342, y=255) -> (x = y?=w337:bool)
                n207 = case shown="真" w337 {
                  tunnel: w340 -> [_ w347]
                  tunnel: w339 -> [_ w346]
                  tunnel: w338 -> [_ w345]
                  frame False {
                  }
                  frame True {
                    n208 = dll-call lib="F:/Bluewave New Energy/SVN_Work/BMS_BootLoader/trunk/BMS_Bootloader/AutoBurn/Settings/ControlCAN.dll" fn="VCI_Transmit"("DeviceType"=w347, "DeviceInd"=w346, "CANInd"=w345, "pSend"=T2 {"ID"=0, "TimeStamp"=0, "TimeFlag"=1, "SendType"=0, "RemoteFlag"=0, "ExternFlag"=0, "DataLen"=1, 1, 0, 0, 0, 0, 0, 0, 0, 0, 0, 0} ("输出簇 2"), "Len"=u32 1) -> ()  [unwired: 5 in, 6 out]
                  }
                }
              }
              frame Enabled {
              }
            }
            n209 = local read "CAN数据"() -> (w331:bool)
            n210 = Enqueue Element(queue=w336, element=w334, error in (no error)=w333) -> (queue out=w335:refnum<queue>, error out=w332:errorcluster)  [unwired: 1 in, 1 out]
            n211 = Not(x=w331) -> (.not. x?=w330:bool)
            n212 = local write "CAN数据"(w330) -> ()
          }
        }
      }
    }
  }
  n213 = while {
    tunnel: w1 -> [w348]
    tunnel: w20 -> [w350]
    tunnel: w1 -> [_]
    stop <- "停止" stop-if-true
    n214 = event shown="[0] 超时" {
      selector: _ -> [_ _ _ _ _ _ _ _ _ _ _]
      dyn-events: _ -> [_ _ _ _ _ _ _ _ _ _ _]
      timeout: 200 -> [_ _ _ _ _ _ _ _ _ _ _]
      tunnel: w348 -> [_ w465 _ _ w525 _ _ _ _ _ _]
      tunnel: w350 -> [_ _ _ _ _ _ _ _ w638 _ _]
      event Timeout {
        n215 = event-data() -> ()  [unwired: 1 in, 2 out]
        n216 = local read "开始下载数据"() -> (w359:bool)
        n217 = local read "update flag"() -> (w360:bool)
        n218 = case shown="真" w360 {
          frame False {
          }
          frame True {
            n219 = local read "start"() -> (w393:u32)
            n220 = Tick Count (ms)() -> (millisecond timer value=w394:u32)
            n221 = Subtract(x=w394, y=w393) -> (x-y=w392:u32)
            n222 = local read "目标板类型"() -> (w390:enum16{"BCU/主板", "BMU/从板"})
            n223 = Divide(x=w392, y=u32 1000) -> (x/y=w389:dbl)
            "耗时：" <- w389
            n224 = To Unsigned Long Integer(number=w389) -> (unsigned 32bit integer=w388:u32)
            n225 = case shown="\"BMU/从板\"" w390 {
              tunnel: w388 -> [w397 w413]
              frame "BCU/主板", Default {
                n226 = Equal?(x=w397, y=80.0) -> (x = y?=w395:bool)
                n227 = case shown="真" w395 {
                  frame False {
                  }
                  frame True {
                    n228 = local read "Info："() -> (w399:string)
                    n229 = local write "update flag"(FALSE ("update flag")) -> ()
                    n230 = Concatenate Strings(w399, "超时请重试" ("字符串")) -> (w400:string)
                    n231 = local write "Info："(w400) -> ()
                    n232 = flat-sequence {
                      frame #0 {
                        n233 = local read "设备索引"() -> (w408:u32)
                        n234 = local read "CAN路数"() -> (w406:u32)
                        n235 = local read "波特率"() -> (w407:T1)
                        n236 = local read "滤波方式"() -> (w405:u8)
                        n237 = local read "工作方式"() -> (w404:u8)
                        n238 = local read "类型"() -> (w409:u32)
                        n239 = call "CAN_Init.vi"("设备类型"=w409, "设备索引"=w408, "波特率"=w407, "CAN路数"=w406, "操作类型"=enum16{"初始化CAN", "关闭CAN"}."关闭CAN", "滤波方式"=w405, "工作方式"=w404) -> ()  [unwired: 11 in, 2 out]
                        n240 = Wait (ms)(milliseconds to wait=u32 2000 ("等待时间（毫秒）")) -> ()  [unwired: 1 out]
                      }
                      frame #1 {
                        n241 = Quit LabVIEW(quit? (T)=TRUE ("退出？(T)")) -> ()
                      }
                    }
                  }
                }
              }
              frame "BMU/从板" {
                n242 = Equal?(x=w413, y=50.0) -> (x = y?=w411:bool)
                n243 = case shown="真" w411 {
                  frame False {
                  }
                  frame True {
                    n244 = local read "Info："() -> (w415:string)
                    n245 = local write "update flag"(FALSE ("update flag")) -> ()
                    n246 = Concatenate Strings(w415, "超时请重试\n" ("字符串")) -> (w416:string)
                    n247 = local write "Info："(w416) -> ()
                    n248 = flat-sequence {
                      frame #0 {
                        n249 = local read "设备索引"() -> (w424:u32)
                        n250 = local read "CAN路数"() -> (w422:u32)
                        n251 = local read "波特率"() -> (w423:T1)
                        n252 = local read "滤波方式"() -> (w421:u8)
                        n253 = local read "工作方式"() -> (w420:u8)
                        n254 = local read "类型"() -> (w425:u32)
                        n255 = call "CAN_Init.vi"("设备类型"=w425, "设备索引"=w424, "波特率"=w423, "CAN路数"=w422, "操作类型"=enum16{"初始化CAN", "关闭CAN"}."关闭CAN", "滤波方式"=w421, "工作方式"=w420) -> ()  [unwired: 11 in, 2 out]
                        n256 = Wait (ms)(milliseconds to wait=u32 2000 ("等待时间（毫秒）")) -> ()  [unwired: 1 out]
                      }
                      frame #1 {
                        n257 = Quit LabVIEW(quit? (T)=TRUE ("退出？(T)")) -> ()
                      }
                    }
                  }
                }
              }
            }
          }
        }
        n258 = case shown="真" w359 {
          frame False {
          }
          frame True {
            n259 = local read "开始下载数据"() -> (w373:u32)
            n260 = Tick Count (ms)() -> (millisecond timer value=w374:u32)
            n261 = Subtract(x=w374, y=w373) -> (x-y=w372:u32)
            n262 = Divide(x=w372, y=u32 1000) -> (x/y=w368:dbl)
            n263 = To Unsigned Long Integer(number=w368) -> (unsigned 32bit integer=w367:u32)
            n264 = Equal?(x=w367, y=3.0) -> (x = y?=w369:bool)
            n265 = case shown="真" w369 {
              frame False {
              }
              frame True {
                n266 = flat-sequence {
                  frame #0 {
                    n267 = local read "Info："() -> (w377:string)
                    n268 = local write "update flag"(FALSE ("update flag")) -> ()
                    n269 = Concatenate Strings(w377, "数据传输中断！\n" ("字符串")) -> (w376:string)
                    n270 = local write "Info："(w376) -> ()
                  }
                  frame #1 {
                  }
                  frame #2 {
                    n271 = local read "设备索引"() -> (w385:u32)
                    n272 = local read "CAN路数"() -> (w383:u32)
                    n273 = local read "波特率"() -> (w384:T1)
                    n274 = local read "滤波方式"() -> (w382:u8)
                    n275 = local read "工作方式"() -> (w381:u8)
                    n276 = local read "类型"() -> (w386:u32)
                    n277 = call "CAN_Init.vi"("设备类型"=w386, "设备索引"=w385, "波特率"=w384, "CAN路数"=w383, "操作类型"=enum16{"初始化CAN", "关闭CAN"}."关闭CAN", "滤波方式"=w382, "工作方式"=w381) -> ()  [unwired: 11 in, 2 out]
                    n278 = Wait (ms)(milliseconds to wait=u32 2000 ("等待时间（毫秒）")) -> ()  [unwired: 1 out]
                  }
                  frame #3 {
                    n279 = Quit LabVIEW(quit? (T)=TRUE ("退出？(T)")) -> ()
                  }
                }
              }
            }
          }
        }
        n280 = local read "boot模式应答...成功"() -> (w363:bool)
        n281 = local read "进入烧录"() -> (w361:bool)
        n282 = local read "boot模式应答计数"() -> (w366:i32)
        n283 = Increment(x=w366) -> (x+1=w354:i32)
        n284 = Equal?(x=w354, y=7) -> (x = y?=w353:bool)
        n285 = Equal?(x=25.0, y=w354) -> (x = y?=w352:bool)
        n286 = Equal?(x=w354, y=25) -> ()  [unwired: 1 out]
        n287 = Equal?(x=35 ("y"), y=w354) -> ()  [unwired: 1 out]
        n288 = Not(x=w363) -> (.not. x?=w362:bool)
        n289 = Compound Arithmetic op=OR(w353, w352) -> (w357:bool)
        n290 = local write "boot模式应答计数"(w354) -> ()
        n291 = Compound Arithmetic op=AND(w357, w362, w361) -> (w364:bool)
        "?" <- w364
        n292 = case shown="真" w364 {
          frame False {
          }
          frame True {
            n293 = local read "目标板类型"() -> (w428:enum16{"BCU/主板", "BMU/从板"})
            n294 = case shown="\"BMU/从板\"" w428 {
              tunnel: [u16 0 ("请选择板号") w440] -> w427
              frame "BCU/主板", Default {
              }
              frame "BMU/从板" {
                n295 = local read "请选择板号"() -> (w440:u16)
              }
            }
            n296 = Multiply(x=w427, y=u16 256) -> (x*y=w431:u16)
            n297 = Add(x=u32 65681 ("ID"), y=w431) -> (x+y=w429:u32)
            n298 = local read "VCI_CAN_OBJ_T"() -> (w433:T2)
            n299 = case shown="1, 默认" w427 {
              tunnel: [w445 w457] -> w437
              tunnel: w433 -> [w444 w456]
              tunnel: w429 -> [w442 w454]
              frame 0 {
                w441 = u8 170
                w448 = u8 0 ("元素")
                n300 = Bundle(cluster=w444, "ID"=w442, "TimeStamp"=u8 0 ("RemoteFlag"), "TimeFlag"=u8 1, "SendType"=u8 0 ("DataLen"), "RemoteFlag"=u8 0, "ExternFlag"=u8 1, "DataLen"=u8 8, u8 1 ("元素"), w441, w441, w441, w441, w448, w448, w448) -> (w445:T2)  [unwired: 3 in]
              }
              frame 1, Default {
                w453 = u8 187
                w460 = u8 0 ("元素")
                n301 = Bundle(cluster=w456, "ID"=w454, "TimeStamp"=u8 0 ("RemoteFlag"), "TimeFlag"=u8 1, "SendType"=u8 0 ("DataLen"), "RemoteFlag"=u8 0, "ExternFlag"=u8 1, "DataLen"=u8 8, u8 1 ("元素"), w453, w453, w453, w453, w460, w460, w460) -> (w457:T2)  [unwired: 3 in]
              }
            }
            n302 = local read "设备索引"() -> (w435:u32)
            n303 = local read "CAN路数"() -> (w434:u32)
            n304 = local read "类型"() -> (w436:u32)
            n305 = dll-call lib="F:/Bluewave New Energy/SVN_Work/BMS_BootLoader/trunk/BMS_Bootloader/AutoBurn/Settings/ControlCAN.dll" fn="VCI_Transmit"("DeviceType"=w436, "DeviceInd"=w435, "CANInd"=w434, "pSend"=w437, "Len"=u32 1) -> ()  [unwired: 5 in, 6 out]
          }
        }
      }
      event "开始监控": Value Change {
        n306 = event-data() -> ("NewVal"=w469:bool)  [unwired: 1 in, 5 out]
        n307 = local write "TEMP"(w469) -> ()
        n308 = local read "通信端口:"() -> (w466:u32)
        n309 = local read "CANET地址格式如：192.168.0.178"() -> (w468:string)
        n310 = local read "设备索引"() -> (w471:u32)
        n311 = local read "CAN路数"() -> (w473:u32)
        n312 = local read "波特率"() -> (w472:T1)
        n313 = local read "滤波方式"() -> (w474:u8)
        n314 = local read "工作方式"() -> (w475:u8)
        n315 = local read "类型"() -> (w470:u32)
        n316 = local read "PC端-协议类型 2"() -> (w467:enum16{"TCP服务器Server", "TCP客户端Client"})
        n317 = case shown="真" w469 {
          tunnel: w470 -> [w494 w518]
          tunnel: w471 -> [w493 w517]
          tunnel: w472 -> [w492 w516]
          tunnel: w473 -> [w491 w515]
          tunnel: w474 -> [w489 w513]
          tunnel: w475 -> [w488 w512]
          tunnel: w468 -> [w482 w510]
          tunnel: w467 -> [w481 w509]
          tunnel: w466 -> [w480 w508]
          tunnel: w465 -> [w479 _]
          frame True {
            w476 = T3."Enabled" ("禁用")
            w484 = "" ("布尔文本.文本")
            w485 = cluster{u32, u32}[] [{0, 0}] ("颜色[4]")
            w486 = FALSE
            n318 = call "CAN_Init.vi"("设备类型"=w494, "设备索引"=w493, "波特率"=w492, "CAN路数"=w491, "操作类型"=enum16{"初始化CAN", "关闭CAN"}."初始化CAN", "error in (no error)"=w479, "滤波方式"=w489, "IP"=w482, "port"=w480, "工作方式"=w488, "PC端-协议类型"=w481) -> ("CAN 操作结果"=w477:bool, "error out"=w478:errorcluster)  [unwired: 7 in]
            n319 = local write "Monitor_flag"(FALSE ("Monitor_flag")) -> ()
            n320 = invoke on="Monitor" class="Bool" method="Reinit To Default"(error in=w478) -> ()  [unwired: 2 in, 3 out]
            n321 = local write "进度"(u8 0 ("进度")) -> ()
            n322 = local write "CAN状态"(w477) -> ()
            n323 = local write "连接状态"(w477) -> ()
            n324 = local write "擦除完成"(w486) -> ()
            n325 = local write "进入烧录模式"(w486) -> ()
            n326 = property on="烧录结果" class="Bool (严格)"("Colors [4]"=w485, "BoolText.Text"=w484) -> ()  [unwired: 2 in, 2 out]
            n327 = property on="校验" class="Bool (严格)"("Colors [4]"=w485, "BoolText.Text"=w484) -> ()  [unwired: 2 in, 2 out]
            n328 = local write "烧录结果"(w486) -> ()
            n329 = case shown="真" w477 {
              frame True {
                n330 = local read "Info："() -> (w495:string)
                n331 = Concatenate Strings(w495, "启动CAN成功.." ("字符串"), "\n") -> (w498:string)
                n332 = local write "Info："(w498) -> ()
              }
              frame False {
                n333 = local read "Info："() -> (w499:string)
                n334 = Concatenate Strings(w499, "启动CAN失败.." ("字符串"), "\n") -> (w502:string)
                n335 = local write "Info："(w502) -> ()
              }
            }
            n336 = property on="手动进入编程模式" class="Bool (严格)"("DisabledEnum"=w476) -> ()  [unwired: 2 in, 2 out]
            n337 = property on="中止编程模式 2" class="Bool (严格)"("DisabledEnum"=w476) -> ()  [unwired: 2 in, 2 out]
          }
          frame False {
            w503 = T3."Disabled and Grayed Out" ("禁用")
            w511 = FALSE ("CAN状态")
            n338 = call "CAN_Init.vi"("设备类型"=w518, "设备索引"=w517, "波特率"=w516, "CAN路数"=w515, "操作类型"=enum16{"初始化CAN", "关闭CAN"}."关闭CAN", "滤波方式"=w513, "IP"=w510, "port"=w508, "工作方式"=w512, "PC端-协议类型"=w509) -> ()  [unwired: 8 in, 2 out]
            n339 = local write "CAN状态"(w511) -> ()
            n340 = local write "连接状态"(w511) -> ()
            n341 = property on="手动进入编程模式" class="Bool (严格)"("DisabledEnum"=w503) -> ()  [unwired: 2 in, 2 out]
            n342 = property on="中止编程模式" class="Bool (严格)"("DisabledEnum"=w503) -> ()  [unwired: 2 in, 2 out]
            n343 = Concatenate Strings("" ("字符串"), "关闭CAN成功..." ("字符串"), "\n") -> (w507:string)
            n344 = local write "Info："(w507) -> ()
          }
        }
      }
      event "Info：": Shortcut Menu Selection (User) {
        n345 = event-data() -> ("ItemPath"=w519:string)  [unwired: 1 in, 7 out]
        n346 = case shown="\"清空\"" w519 {
          frame "假", Default {
          }
          frame "清空" {
            n347 = local write "Info："("" ("Info：")) -> ()
          }
        }
      }
      event Menu Selection (User) {
        n348 = event-data() -> ("ItemTag"=w522:string)  [unwired: 1 in, 6 out]
        n349 = case shown="\"烧录多块\"" w522 {
          tunnel: [FALSE ("Mode") TRUE ("Mode")] -> w521
          frame "烧录多块" {
          }
          frame "烧录一块", Default {
          }
        }
        n350 = local write "Mode"(w521) -> ()
      }
      event "类型": Value Change {
        n351 = event-data() -> ("NewVal"=w526:u32)  [unwired: 1 in, 5 out]
        n352 = case shown="17" w526 {
          tunnel: w525 -> [_ w530]
          frame 0, Default {
          }
          frame 17 {
            n353 = call "PortSet.vi"("error in (no error)"=w530) -> ("PC端-协议类型 2"=→"PC端-协议类型 2":enum16{"TCP服务器Server", "TCP客户端Client"}, "通信端口:"=→"通信端口:":dbl, "CANET地址格式如：192.168.0.178"=→"CANET地址格式如：192.168.0.178":string)  [unwired: 7 in, 1 out]
          }
        }
      }
      event "类型": Mouse Down {
        w531 = u16 4 items=["PCI5121"=1, "PCI9810"=2, "USBCAN1"=3, "USBCAN2"=4, "PCI9820"=5, "CAN232"=6, "PCI5110"=7, "CANLite(mini)"=8, "ISA9620"=9, "ISA5420"=10, "PC104CAN"=11, "CANET"=17, "DNP9810"=13] ("设备类型")
        n354 = event-data() -> ()  [unwired: 1 in, 8 out]
        n355 = local write "类型"(w531) -> ()
      }
      event "Monitor": Value Change {
        n356 = event-data() -> ("NewVal"=w535:bool)  [unwired: 1 in, 5 out]
        n357 = local read "板类型"() -> (w534:enum16{"请选择板类型", "主板", "从板", "高压板"})
        n358 = Equal?(x=w534, y=enum16{"请选择板类型", "主板", "从板", "高压板"}."请选择板类型") -> (x = y?=w532:bool)
        n359 = case shown="真" w532 {
          tunnel: w535 -> [w538 _]
          frame False {
            n360 = Select(t=0.0, s=w538, f=2.0) -> (s? t:f=w539:dbl)
            n361 = property on="手动进入编程模式" class="Bool (严格)"("Disabled"=w539) -> ()  [unwired: 2 in, 2 out]
            "Monitor_flag" <- w538
          }
          frame True {
            n362 = invoke on="Monitor" class="Bool" method="Reinit To Default"() -> ()  [unwired: 3 in, 3 out]
            n363 = One Button Dialog(message=" 请选择板的类型！！" ("消息")) -> ()  [unwired: 1 in, 1 out]
          }
        }
      }
      event "应用程序路径": Value Change {
        n364 = event-data() -> ("NewVal"=w542:path)  [unwired: 1 in, 5 out]
        n365 = Not A Number/Path/Refnum?(number/path/refnum=w542) -> (NaN/Path/Refnum?=w545:bool)
        n366 = Strip Path(path=w542) -> (name=w541:string)  [unwired: 1 out]
        n367 = String Subset(string=w541, offset (0)=6 ("偏移量(0)"), length (rest)=2 ("长度（剩余）")) -> (substring=w546:string)
        n368 = case shown="\"SS\"" w546 {
          tunnel: [TRUE ("y") FALSE ("y") FALSE ("y")] -> w543
          frame "假", Default {
            n369 = local read "Info："() -> (w550:string)
            n370 = Concatenate Strings(w550, "无法识别板类型！\n" ("字符串")) -> (w552:string)
            n371 = local write "Info："(w552) -> ()
          }
          frame "MS" {
            n372 = local read "Info："() -> (w554:string)
            n373 = local write "目标板类型"(enum16{"BCU/主板", "BMU/从板"}."BCU/主板" ("类型")) -> ()
            n374 = property on="请选择板号" class="Ring (严格)"("Visible"=FALSE ("可见")) -> ()  [unwired: 2 in, 2 out]
            n375 = Concatenate Strings(w554, "通过文件识别为主板！\n" ("字符串")) -> (w555:string)
            n376 = local write "Info："(w555) -> ()
          }
          frame "SS" {
            n377 = local read "Info："() -> (w560:string)
            n378 = local write "目标板类型"(enum16{"BCU/主板", "BMU/从板"}."BMU/从板" ("类型")) -> ()
            n379 = property on="请选择板号" class="Ring (严格)"("Visible"=TRUE ("可见")) -> ()  [unwired: 2 in, 2 out]
            n380 = Concatenate Strings(w560, "通过文件识别为从板！\n" ("字符串")) -> (w561:string)
            n381 = local write "Info："(w561) -> ()
          }
        }
        n382 = Or(x=w545, y=w543) -> (x .or. y?=w544:bool)
        n383 = case shown="假" w544 {
          tunnel: w542 -> [w600 _]
          frame False {
            n384 = Path To String(path=w600) -> (string=w574:string)
            n385 = local read "Info："() -> (w570:string)
            n386 = String Subset(string=w574, offset (0)=6 ("偏移量(0)"), length (rest)=2 ("长度（剩余）")) -> (substring=w571:string)
            n387 = call-poly <vilib>:"Read From Spreadsheet File.vi"("file path (dialog if empty)"=w600) -> ("all rows"=w602:string[][])  [unwired: 6 in, 4 out]
            n388 = call <vilib>:"Space Constant.vi"() -> ("String"=w598:string)
            n389 = Search and Replace String(replace all?=TRUE ("替换全部？(F)"), input string=w574, search string=w598, replace string="" ("替换字符串(\"\")")) -> (result string=w585:string)  [unwired: 4 in, 3 out]
            n390 = case shown="\"真\"" w571 {
              frame "假", Default {
              }
              frame "真" {
              }
            }
            n391 = Concatenate Strings(w570, "文件加载成功！\n" ("字符串")) -> (w568:string)
            n392 = Index Array(array=w602, index (col)=0 ("禁用的索引 (列)")) -> (element=w589:string[])  [unwired: 1 in]
            n393 = Search/Split String(string=w585, search string/char (-)="(MD5=" ("搜索字符串/字符(-)")) -> (match + rest of string=w582:string, offset of match=w592:i32)  [unwired: 1 in, 1 out]
            n394 = local write "Info："(w568) -> ()
            n395 = Delete From Array(array=w589, length=1 ("长度"), index=0 ("索引")) -> (array with subset deleted=w581:string[])  [unwired: 1 out]
            n396 = call <vilib>:"MD5Checksum File.vi"("Path"=w600) -> ("MD5 message-digest"=w565:string)  [unwired: 9 in, 1 out]
            n397 = Array Size(array=w581) -> (size(s)=w579:i32)
            n398 = Decrement(x=w579) -> (x-1=w578:i32)
            n399 = Delete From Array(array=w581, length=1 ("长度"), index=w578) -> (array with subset deleted=w576:string[])  [unwired: 1 out]
            n400 = Array Size(array=w576) -> (size(s)=→"总行数":i32)
            n401 = local write "校验码实际值"(w565) -> ()
            n402 = Add(x=w592, y=5) -> (x+y=w593:i32)
            n403 = Search/Split String(string=w585, search string/char (-)=")" ("搜索字符串/字符(-)")) -> ()  [unwired: 1 in, 3 out]
            n404 = String Subset(string=w582, offset (0)=45 ("偏移量(0)"), length (rest)=8 ("长度（剩余）")) -> ()  [unwired: 1 out]
            n405 = String Subset(string=w585, offset (0)=w593, length (rest)=32 ("长度（剩余）")) -> (substring=w583:string)
            n406 = Equal?(x=w583, y=w565) -> (x = y?=w590:bool)
            n407 = case shown="真" w590 {
              frame False {
                n408 = Build Array(cluster{u32, u32} {16711680, 0}) -> (w632:cluster{u32, u32}[])
                n409 = property on="MD5校验" class="Bool (严格)"("Colors [4]"=w632, "BoolText.Text"="失败" ("布尔文本.文本")) -> ()  [unwired: 2 in, 2 out]
              }
              frame True {
                n410 = Build Array(cluster{u32, u32} {6618880, 0}) -> (w635:cluster{u32, u32}[])
                n411 = property on="MD5校验" class="Bool (严格)"("Colors [4]"=w635, "BoolText.Text"="成功" ("布尔文本.文本")) -> ()  [unwired: 2 in, 2 out]
              }
            }
            n412 = local write "校验码期望值"(w583) -> ()
            n413 = for {
              tunnel: w576 -> [w613] mode=indexing
              shift-right: [w611] -> w566
              shift-left: u16 0 ("偏移量(0)") -> [w612]
              tunnel: [w605] -> w567 mode=indexing
              n414 = String Subset(string=w613, offset (0)=1 ("偏移量(0)"), length (rest)=1 ("长度（子字符串长度）")) -> (substring=w616:string)
              n415 = case shown="\"1\", 默认" w616 {
                tunnel: ["01" ("子字符串(\"\")") "02" ("子字符串(\"\")")] -> w617
                frame "1", Default {
                }
                frame "2" {
                }
              }
              n416 = String Subset(string=w613, offset (0)=2 ("偏移量(0)")) -> (substring=w619:string)  [unwired: 1 in]
              n417 = Concatenate Strings("FFFFFFFFFFFF" ("子字符串(\"\")"), w617, w619) -> (w605:string)
              n418 = String Subset(string=w605, offset (0)=12 ("偏移量(0)")) -> (substring=w603:string)  [unwired: 1 in]
              n419 = String Length(string=w603) -> (length=w610:i32)
              n420 = Divide(x=w610, y=2) -> (x/y=w608:dbl)
              n421 = for {
                N: w608 -> [_]
                tunnel: w603 -> [w628]
                shift-right: [w623] -> w606
                shift-left: u16 0 ("偏移量(0)") -> [w621]
                i -> [w627]
                w625 = 2 ("x")
                n422 = Multiply(x=w625, y=w627) -> (x*y=w626:i32)
                n423 = String Subset(string=w628, offset (0)=w626, length (rest)=w625) -> (substring=w624:string)
                n424 = call "ASCII_To_Hex.vi"("ASCII String"=w624) -> ("hex1"=w622:u8)  [unwired: 6 in, 4 out]
                n425 = Add(x=w621, y=w622) -> (x+y=w623:u16)
              }
              n426 = Add(x=w612, y=w606) -> (x+y=w611:u16)
            }
            n427 = local write "CRC16"(w566) -> ()
            n428 = local write "子数组"(w567) -> ()
          }
          frame True {
          }
        }
      }
      event "手动进入编程模式": Value Change {
        n429 = event-data() -> ("NewVal"=w637:bool)  [unwired: 1 in, 5 out]
        n430 = case shown="真" w637 {
          tunnel: w638 -> [_ w641]
          frame False {
          }
          frame True {
            n431 = Empty String/Path?(string/path="应用程序路径") -> (empty?=w639:bool)
            n432 = case shown="假" w639 {
              tunnel: w641 -> [w645 _]
              frame False {
                n433 = local write "update flag"(TRUE ("update flag")) -> ()
                n434 = Two Button Dialog(message="请确认需要下载的BMU编号正确！\nBMU正常上电！\n应用程序文件选择正确 !" ("消息")) -> (T button?=w644:bool)  [unwired: 2 in]
                n435 = case shown="真" w644 {
                  tunnel: w645 -> [_ w646]
                  frame False {
                  }
                  frame True {
                    n436 = stacked-sequence {
                      tunnel: w646 -> [_ _ _]
                      frame #0 {
                        n437 = disable-structure shown="启用" {
                          frame Enabled {
                            n438 = local read "CAN路数"() -> (w652:u32)
                            n439 = local read "设备索引"() -> (w653:u32)
                            n440 = local read "类型"() -> (w654:u32)
                            n441 = dll-call lib="F:/Bluewave New Energy/SVN_Work/BMS_BootLoader/trunk/BMS_Bootloader/AutoBurn/Settings/ControlCAN.dll" fn="VCI_ClearBuffer" label="VCI_Clearbuffer"(error in=errorcluster {"status"=FALSE, "code"=0, "source"=""} ("错误输入（无错误）"), "DeviceType"=w654, "DeviceInd"=w653, "CANInd"=w652) -> (error out=→"错误输出 3":errorcluster)  [unwired: 3 in, 4 out]
                          }
                          frame Disabled {
                          }
                        }
                        n442 = local write "boot模式应答...成功"(FALSE) -> ()
                        "boot模式应答计数" <- 0
                        "进入烧录" <- TRUE ("布尔")
                      }
                      frame #1 {
                        w660 = TRUE ("T1")
                        w659 = TRUE ("T1")
                        n443 = Concatenate Strings("" ("字符串"), "boot模式请求..." ("字符串"), "\n") -> (w658:string)
                        n444 = local write "Info："(w658) -> ()
                        n445 = local write "T2"(w659) -> ()
                        n446 = local write "T3"(w660) -> ()
                        n447 = local write "T1"(w659) -> ()
                        n448 = local write "T4"(w660) -> ()
                        n449 = local write "T5"(w660) -> ()
                        n450 = local write "T6"(w660) -> ()
                        n451 = local write "T7"(w660) -> ()
                        n452 = local write "T8"(u8 0 ("T8")) -> ()
                        n453 = local write "T9"(w660) -> ()
                      }
                      frame #2 {
                        n454 = local read "目标板类型"() -> (w663:enum16{"BCU/主板", "BMU/从板"})
                        n455 = case shown="\"BMU/从板\"" w663 {
                          tunnel: [u16 0 ("请选择板号") w676] -> w664
                          frame "BCU/主板", Default {
                          }
                          frame "BMU/从板" {
                            n456 = local read "请选择板号"() -> (w676:u16)
                          }
                        }
                        n457 = Tick Count (ms)() -> (millisecond timer value=→"start":u32)
                        n458 = Multiply(x=w664, y=u16 256) -> (x*y=w667:u16)
                        n459 = Add(x=u32 65681 ("ID"), y=w667) -> (x+y=w665:u32)
                        n460 = local read "VCI_CAN_OBJ_T"() -> (w669:T2)
                        n461 = case shown="1, 默认" w664 {
                          tunnel: [w681 w693] -> w673
                          tunnel: w669 -> [w680 w692]
                          tunnel: w665 -> [w678 w690]
                          frame 0 {
                            w677 = u8 170
                            w684 = u8 0 ("元素")
                            n462 = Bundle(cluster=w680, "ID"=w678, "TimeStamp"=u8 0 ("RemoteFlag"), "TimeFlag"=u8 1, "SendType"=u8 0 ("DataLen"), "RemoteFlag"=u8 0, "ExternFlag"=u8 1, "DataLen"=u8 8, u8 1 ("元素"), w677, w677, w677, w677, w684, w684, w684) -> (w681:T2)  [unwired: 3 in]
                          }
                          frame 1, Default {
                            w689 = u8 187
                            w696 = u8 0 ("元素")
                            n463 = Bundle(cluster=w692, "ID"=w690, "TimeStamp"=u8 0 ("RemoteFlag"), "TimeFlag"=u8 1, "SendType"=u8 0 ("DataLen"), "RemoteFlag"=u8 0, "ExternFlag"=u8 1, "DataLen"=u8 8, u8 1 ("元素"), w689, w689, w689, w689, w696, w696, w696) -> (w693:T2)  [unwired: 3 in]
                          }
                        }
                        n464 = local read "设备索引"() -> (w671:u32)
                        n465 = local read "CAN路数"() -> (w670:u32)
                        n466 = local read "类型"() -> (w672:u32)
                        n467 = dll-call lib="F:/Bluewave New Energy/SVN_Work/BMS_BootLoader/trunk/BMS_Bootloader/AutoBurn/Settings/ControlCAN.dll" fn="VCI_Transmit"("DeviceType"=w672, "DeviceInd"=w671, "CANInd"=w670, "pSend"=w673, "Len"=u32 1) -> ()  [unwired: 5 in, 6 out]
                      }
                    }
                  }
                }
              }
              frame True {
                n468 = One Button Dialog(message="请先选择应用程序路径" ("消息")) -> ()  [unwired: 1 in, 1 out]
              }
            }
          }
        }
      }
      event "开始监控 2": Value Change {
        n469 = event-data() -> ("NewVal"=w702:bool)  [unwired: 1 in, 5 out]
        n470 = local write "TEMP"(w702) -> ()
      }
      event Panel Close? {
        n471 = event-data() -> ()  [unwired: 1 in, 4 out]
        n472 = local read "设备索引"() -> (w705:u32)
        n473 = local read "CAN路数"() -> (w707:u32)
        n474 = local read "波特率"() -> (w706:T1)
        n475 = local read "滤波方式"() -> (w708:u8)
        n476 = local read "工作方式"() -> (w709:u8)
        n477 = local read "类型"() -> (w704:u32)
        n478 = call "CAN_Init.vi"("设备类型"=w704, "设备索引"=w705, "波特率"=w706, "CAN路数"=w707, "操作类型"=enum16{"初始化CAN", "关闭CAN"}."关闭CAN", "滤波方式"=w708, "工作方式"=w709) -> ("error out"=w703:errorcluster)  [unwired: 11 in, 1 out]
        n479 = flat-sequence {
          tunnel: w703 -> [_]
          frame #0 {
            n480 = Quit LabVIEW(quit? (T)=TRUE ("退出？(T)")) -> ()
          }
        }
        n481 = event-data("Discard?"=TRUE ("放弃？")) -> ()  [unwired: 1 in, 1 out]
      }
    }
  }
  n482 = while {
    tunnel: w20 -> [w717]
    shift-right: [w720] -> _
    shift-left: w33 -> [w721]
    shift-right: [w718] -> _
    shift-left: "" -> [w719]
    tunnel: w7 -> [w716]
    stop <- "停止 3" stop-if-true
    n483 = local read "update flag"() -> (w713:bool)
    n484 = Dequeue Element(queue=w717, error in (no error)=w716) -> (element=w714:T2, error out=w715:errorcluster)  [unwired: 1 in, 2 out]
    n485 = case shown="真" w713 {
      tunnel: w721 -> [_ w740]
      tunnel: [_ w739] -> w720
      tunnel: w719 -> [_ w738]
      tunnel: [_ w737] -> w718
      tunnel: w717 -> [_ w735]
      tunnel: w715 -> [_ w734]
      tunnel: w714 -> [_ w733]
      frame False {
      }
      frame True {
        n486 = local read "VCI_CAN_OBJ_T"() -> (w743:T2)
        n487 = local read "CAN路数"() -> (w741:u32)
        n488 = Unbundle(w733) -> ("ID"=w732:u32, w731:u8, w730:u8, w729:u8, w728:u8, w727:u8, w726:u8, w725:u8, w724:u8)  [unwired: 9 out]
        n489 = local read "类型"() -> (w742:u32)
        n490 = local read "设备索引"() -> (w723:u32)
        n491 = case shown="19100..19120, 191FF" w732 {
          selector: w732 -> [_ w939 w1021 w1077 w1265 _ _ _ _ w2008]
          tunnel: w733 -> [_ _ _ _ _ _ _ _ _ _]
          tunnel: w743 -> [w757 _ _ w1081 w1269 w1487 w1552 _ w1788 _]
          tunnel: w742 -> [w756 _ _ w1080 w1268 w1486 w1554 w1682 w1796 _]
          tunnel: w723 -> [w755 _ _ w1079 w1267 w1485 w1553 w1681 w1795 _]
          tunnel: w741 -> [w754 _ _ w1078 w1266 w1484 w1551 w1680 w1794 _]
          tunnel: w740 -> [w753 _ _ _ _ w1483 w1556 w1679 w1790 w2010]
          tunnel: [w753 _ _ _ _ w1483 w1555 w1679 w1791 w2010] -> w739
          tunnel: w738 -> [w752 _ _ _ _ w1482 w1550 w1684 w1792 w2009]
          tunnel: [w752 _ _ _ _ w1482 w1549 w1683 w1793 w2009] -> w737
          tunnel: "板类型" -> [_ _ _ _ _ _ w1548 w1678 w1789 _]
          tunnel: w735 -> [_ _ _ _ _ w1481 w1547 w1677 w1787 _]
          tunnel: w734 -> [_ _ _ _ _ _ _ _ _ _]
          tunnel: w733 -> [_ _ _ _ _ _ _ w1668 _ _]
          tunnel: w733 -> [_ _ _ _ _ _ _ _ w1786 _]
          tunnel: w731 -> [w751 w942 w1023 w1084 _ _ _ _ _ _]
          tunnel: w730 -> [w750 w937 _ _ _ _ _ _ _ _]
          tunnel: w729 -> [w749 w936 _ _ w1263 _ _ _ _ _]
          tunnel: w728 -> [w748 w935 _ _ _ _ _ _ _ _]
          tunnel: w727 -> [w747 w934 _ _ _ _ _ _ _ _]
          tunnel: w726 -> [w746 _ _ _ _ _ _ _ _ _]
          tunnel: w725 -> [w745 _ _ _ _ _ _ _ _ w2004]
          tunnel: w724 -> [w744 _ _ _ _ _ _ _ _ w2003]
          frame 4 {
            (unwired) TRUE
            n492 = disable-structure shown="禁用" {
              disable-tunnel: w757 -> [w769 _]
              disable-tunnel: w756 -> [w768 _]
              disable-tunnel: w755 -> [w767 _]
              disable-tunnel: w754 -> [w766 _]
              disable-tunnel: w751 -> [w765 _]
              disable-tunnel: w750 -> [w764 _]
              disable-tunnel: w749 -> [w763 _]
              disable-tunnel: w748 -> [w762 _]
              disable-tunnel: w747 -> [w761 _]
              disable-tunnel: w746 -> [w760 _]
              disable-tunnel: w745 -> [w759 _]
              disable-tunnel: w744 -> [w758 _]
              frame Disabled {
                n493 = stacked-sequence {
                  tunnel: w769 -> [w794]
                  tunnel: w768 -> [w793]
                  tunnel: w767 -> [w792]
                  tunnel: w766 -> [w791]
                  tunnel: w765 -> [w790]
                  tunnel: w764 -> [w789]
                  tunnel: w763 -> [w788]
                  tunnel: w762 -> [w787]
                  tunnel: w761 -> [w786]
                  tunnel: w760 -> [w785]
                  tunnel: w759 -> [w784]
                  tunnel: w758 -> [w783]
                  frame #0 {
                    n494 = Equal?(x=w790, y=u8 252) -> (x = y?=w774:bool)
                    n495 = Equal?(x=w789, y=u8 7) -> (x = y?=w773:bool)
                    n496 = Equal?(x=w788, y=u8 3) -> (x = y?=w772:bool)
                    n497 = Equal?(x=w787, y=u8 255) -> (x = y?=w771:bool)
                    n498 = Equal?(x=w785, y=u8 0) -> ()  [unwired: 1 out]
                    n499 = Equal?(x=w783, y=u8 1) -> ()  [unwired: 1 out]
                    n500 = Equal?(x=w786, y=u8 0) -> ()  [unwired: 1 out]
                    n501 = Equal?(x=w784, y=u8 0) -> ()  [unwired: 1 out]
                    n502 = Compound Arithmetic op=AND(w774, w773, w772, w771) -> (w770:bool)
                    n503 = case shown="真" w770 {
                      tunnel: w794 -> [_ w802]
                      tunnel: w793 -> [_ w801]
                      tunnel: w792 -> [_ w800]
                      tunnel: w791 -> [_ w799]
                      frame False {
                      }
                      frame True {
                        n504 = local read "T8"() -> (w798:u8)
                        n505 = Increment(x=w798) -> (x+1=w797:u8)
                        n506 = Greater Or Equal?(x=w797, y=u8 10) -> (x >= y?=w795:bool)
                        n507 = local write "T8"(w797) -> ()
                        n508 = case shown="真" w795 {
                          tunnel: w802 -> [_ w812]
                          tunnel: w801 -> [_ w811]
                          tunnel: w800 -> [_ w810]
                          tunnel: w799 -> [_ w809]
                          frame False {
                          }
                          frame True {
                            n509 = local read "子数组"() -> (w808:string[])
                            n510 = local read "Info："() -> (w804:string)
                            n511 = Array Size(array=w808) -> (size(s)=w807:i32)
                            n512 = while {
                              tunnel: w812 -> [w823]
                              tunnel: w811 -> [w822]
                              tunnel: w810 -> [w821]
                              tunnel: w809 -> [w820]
                              tunnel: w808 -> [w819] mode=indexing
                              tunnel: w807 -> [w816]
                              i -> [w817]
                              stop <- w815 stop-if-true
                              n513 = while {
                                tunnel: w823 -> [w839]
                                tunnel: w822 -> [w838]
                                tunnel: w821 -> [w837]
                                tunnel: w820 -> [w836]
                                shift-right: [w831] -> _
                                shift-left: w819 -> [w832]
                                tunnel: w816 -> [w829]
                                tunnel: w817 -> [w825]
                                stop <- w824 stop-if-true
                                n514 = String Length(string=w832) -> (length=w830:i32)
                                n515 = Greater Or Equal?(x=w830, y=8) -> (x >= y?=w833:bool)
                                n516 = case shown="假" w833 {
                                tunnel: w839 -> [w867 w877]
                                tunnel: w838 -> [w866 w876]
                                tunnel: w837 -> [w865 w875]
                                tunnel: w836 -> [w864 w874]
                                tunnel: w832 -> [w853 w873]
                                tunnel: [w841 w872] -> w831
                                tunnel: [FALSE TRUE] -> w824
                                tunnel: w830 -> [_ w870]
                                tunnel: w830 -> [_ w868]
                                frame True {
                                w860 = u8 0 ("元素")
                                n517 = String Subset(string=w853, offset (0)=8 ("偏移量(0)")) -> (substring=w841:string)  [unwired: 1 in]
                                n518 = String Subset(string=w853, length (rest)=8 ("长度（剩余）")) -> (substring=w851:string)  [unwired: 1 in]
                                n519 = String To Byte Array(string=w851) -> (unsigned byte array=w850:u8[])
                                n520 = Index Array(array=w850) -> (element #1=w849:u8, element #2=w848:u8, element #3=w847:u8, element #4=w846:u8, element #5=w845:u8, element #6=w844:u8, element #7=w843:u8, element #8=w842:u8)  [unwired: 8 in]
                                n521 = Bundle(cluster=w867, "ID"=u32 5, "TimeStamp"=u8 0 ("RemoteFlag"), "TimeFlag"=u8 1, "SendType"=u8 0 ("DataLen"), "RemoteFlag"=u8 0, "DataLen"=u8 8, w849, w848, w847, w846, w845, w844, w843, w842, w860, w860, w860) -> (w855:T2)  [unwired: 1 in]
                                n522 = dll-call lib="F:/Bluewave New Energy/SVN_Work/BMS_BootLoader/trunk/BMS_Bootloader/AutoBurn/Settings/ControlCAN.dll" fn="VCI_Transmit"("DeviceType"=w866, "DeviceInd"=w865, "CANInd"=w864, "pSend"=w855, "Len"=u32 1) -> ()  [unwired: 5 in, 6 out]
                                }
                                frame False {
                                n523 = Greater Than 0?(x=w870) -> (x > 0?=w869:bool)
                                n524 = case shown="真" w869 {
                                tunnel: w877 -> [w904 w911]
                                tunnel: w876 -> [w903 w910]
                                tunnel: w875 -> [w902 w909]
                                tunnel: w874 -> [w901 w908]
                                tunnel: w873 -> [w890 _]
                                tunnel: [w879 _] -> w872
                                tunnel: w868 -> [_ w906]
                                frame True {
                                w897 = u8 0 ("元素")
                                n525 = String Subset(string=w890, offset (0)=8 ("偏移量(0)")) -> (substring=w879:string)  [unwired: 1 in]
                                n526 = String Subset(string=w890, length (rest)=8 ("长度（剩余）")) -> (substring=w889:string)  [unwired: 1 in]
                                n527 = String To Byte Array(string=w889) -> (unsigned byte array=w888:u8[])
                                n528 = Index Array(array=w888) -> (element #1=w887:u8, element #2=w886:u8, element #3=w885:u8, element #4=w884:u8, element #5=w883:u8, element #6=w882:u8, element #7=w881:u8, element #8=w880:u8)  [unwired: 8 in]
                                n529 = Bundle(cluster=w904, "ID"=u32 5, "TimeStamp"=u8 0 ("RemoteFlag"), "TimeFlag"=u8 1, "SendType"=u8 0 ("DataLen"), "RemoteFlag"=u8 0, "DataLen"=u8 8, w887, w886, w885, w884, w883, w882, w881, w880, w897, w897, w897) -> (w892:T2)  [unwired: 1 in]
                                n530 = dll-call lib="F:/Bluewave New Energy/SVN_Work/BMS_BootLoader/trunk/BMS_Bootloader/AutoBurn/Settings/ControlCAN.dll" fn="VCI_Transmit"("DeviceType"=w903, "DeviceInd"=w902, "CANInd"=w901, "pSend"=w892, "Len"=u32 1) -> ()  [unwired: 5 in, 6 out]
                                }
                                frame False {
                                n531 = Quotient & Remainder(x=w906, y=8) -> (x-y*floor(x/y)=w905:i32)  [unwired: 1 out]
                                n532 = case shown="0" w905 {
                                tunnel: w911 -> [w933 _]
                                tunnel: w910 -> [w932 _]
                                tunnel: w909 -> [w931 _]
                                tunnel: w908 -> [w930 _]
                                frame 0 {
                                w926 = u8 0 ("元素")
                                n533 = Index Array(array=u8[] [0, 0, 0, 0, 0, 0, 0, 0] ("数组")) -> (element #1=w920:u8, element #2=w919:u8, element #3=w918:u8, element #4=w917:u8, element #5=w916:u8, element #6=w915:u8, element #7=w914:u8, element #8=w913:u8)  [unwired: 8 in]
                                n534 = Bundle(cluster=w933, "ID"=u32 5, "TimeStamp"=u8 0 ("RemoteFlag"), "TimeFlag"=u8 1, "SendType"=u8 0 ("DataLen"), "RemoteFlag"=u8 0, "DataLen"=u8 8, w920, w919, w918, w917, w916, w915, w914, w913, w926, w926, w926) -> (w921:T2)  [unwired: 1 in]
                                n535 = dll-call lib="F:/Bluewave New Energy/SVN_Work/BMS_BootLoader/trunk/BMS_Bootloader/AutoBurn/Settings/ControlCAN.dll" fn="VCI_Transmit"("DeviceType"=w932, "DeviceInd"=w931, "CANInd"=w930, "pSend"=w921, "Len"=u32 1) -> ()  [unwired: 5 in, 6 out]
                                }
                                frame 1, Default {
                                }
                                }
                                }
                                }
                                }
                                }
                                n536 = Divide(x=w825, y=w829) -> (x/y=w828:dbl)
                                n537 = Multiply(x=w828, y=100.0) -> (x*y=w826:dbl)
                                n538 = local write "进度"(w826) -> ()
                                n539 = Wait (ms)(milliseconds to wait=u32 5 ("等待时间（毫秒）")) -> ()  [unwired: 1 out]
                              }
                              n540 = Equal?(x=w817, y=w816) -> (x = y?=w813:bool)
                              n541 = local read "连接状态"() -> (w818:bool)
                              n542 = Not(x=w818) -> (.not. x?=w814:bool)
                              n543 = Or(x=w813, y=w814) -> (x .or. y?=w815:bool)
                            }
                            n544 = Concatenate Strings(w804, "程序下载中.." ("字符串"), "\n") -> (w803:string)
                            n545 = local write "Info："(w803) -> ()
                          }
                        }
                      }
                    }
                  }
                }
              }
              frame Enabled {
              }
            }
          }
          frame 102656..102688, 102911 {
            n546 = To Unsigned Byte Integer(number=w939) -> (unsigned 8bit integer=w938:u8)
            n547 = Equal?(x=w942, y=u8 85) -> (x = y?=w941:bool)
            n548 = case shown="真" w941 {
              tunnel: w938 -> [_ w974]
              tunnel: w937 -> [_ w971]
              tunnel: w936 -> [_ w969]
              tunnel: w935 -> [_ w970]
              tunnel: w934 -> [_ w968]
              frame False {
                n549 = local write "update flag"(FALSE ("update flag")) -> ()
                n550 = flat-sequence {
                  frame #0 {
                    n551 = local read "设备索引"() -> (w955:u32)
                    n552 = local read "CAN路数"() -> (w953:u32)
                    n553 = local read "波特率"() -> (w954:T1)
                    n554 = local read "滤波方式"() -> (w952:u8)
                    n555 = local read "工作方式"() -> (w951:u8)
                    n556 = local read "类型"() -> (w956:u32)
                    n557 = call "CAN_Init.vi"("设备类型"=w956, "设备索引"=w955, "波特率"=w954, "CAN路数"=w953, "操作类型"=enum16{"初始化CAN", "关闭CAN"}."关闭CAN", "滤波方式"=w952, "工作方式"=w951) -> ()  [unwired: 11 in, 2 out]
                    n558 = Wait (ms)(milliseconds to wait=u32 2000 ("等待时间（毫秒）")) -> ()  [unwired: 1 out]
                  }
                  frame #1 {
                    n559 = Quit LabVIEW(quit? (T)=TRUE ("退出？(T)")) -> ()
                  }
                }
                n560 = local read "Info："() -> (w945:string)
                n561 = One Button Dialog(message="程序下载错误，请断电重试！" ("消息")) -> ()  [unwired: 1 in, 1 out]
                n562 = Concatenate Strings(w945, "boot模式应答...失败" ("字符串"), "\n") -> (w948:string)
                n563 = local write "Info："(w948) -> ()
              }
              frame True {
                n564 = Join Numbers(hi=w971, lo=w970) -> ((hi.lo)=w967:u16)
                n565 = Join Numbers(hi=w968, lo=w969) -> ((hi.lo)=w966:u16)
                n566 = Join Numbers(hi=w967, lo=w966) -> ((hi.lo)=w965:u32)
                n567 = Not(x=w965) -> (.not. x?=w964:u32)
                "Random" <- w964
                n568 = Split Number(x=w964) -> (hi(x)=w963:u16, lo(x)=w962:u16)
                n569 = Split Number(x=w963) -> (hi(x)=w961:u8, lo(x)=w960:u8)
                n570 = Split Number(x=w962) -> (hi(x)=w959:u8, lo(x)=w958:u8)
                n571 = stacked-sequence {
                  tunnel: w974 -> [_ w995]
                  tunnel: w961 -> [_ w990]
                  tunnel: w960 -> [_ w989]
                  tunnel: w959 -> [_ w988]
                  tunnel: w958 -> [_ w987]
                  frame #0 {
                    n572 = disable-structure shown="启用" {
                      frame Enabled {
                        n573 = local read "CAN路数"() -> (w982:u32)
                        n574 = local read "设备索引"() -> (w983:u32)
                        n575 = local read "类型"() -> (w984:u32)
                        n576 = dll-call lib="F:/Bluewave New Energy/SVN_Work/BMS_BootLoader/trunk/BMS_Bootloader/AutoBurn/Settings/ControlCAN.dll" fn="VCI_ClearBuffer" label="VCI_Clearbuffer"(error in=errorcluster {"status"=FALSE, "code"=0, "source"=""} ("错误输入（无错误）"), "DeviceType"=w984, "DeviceInd"=w983, "CANInd"=w982) -> (error out=→"错误输出 12":errorcluster)  [unwired: 3 in, 4 out]
                      }
                      frame Disabled {
                      }
                    }
                    n577 = Wait (ms)(milliseconds to wait=u32 1000 ("等待时间（毫秒）")) -> ()  [unwired: 1 out]
                  }
                  frame #1 {
                    w996 = u16 256 ("y")
                    w1011 = u8 0 ("元素")
                    n578 = local read "目标板类型"() -> (w986:enum16{"BCU/主板", "BMU/从板"})
                    n579 = case shown="\"BCU/主板\", 默认" w986 {
                      tunnel: [u16 0 ("请选择板号") w1018] -> w985
                      frame "BCU/主板", Default {
                      }
                      frame "BMU/从板" {
                        n580 = local read "请选择板号"() -> (w1018:u16)
                      }
                    }
                    n581 = local read "设备索引"() -> (w1006:u32)
                    n582 = local read "CAN路数"() -> (w1005:u32)
                    n583 = local read "类型"() -> (w1007:u32)
                    n584 = Multiply(x=w985, y=w996) -> ()  [unwired: 1 out]
                    n585 = Multiply(x=w996, y=w995) -> (x*y=w994:u16)
                    n586 = local read "Info："() -> (w1000:string)
                    n587 = Add(x=u32 131217 ("ID"), y=w994) -> (x+y=w1001:u32)
                    n588 = local read "VCI_CAN_OBJ_T"() -> (w1004:T2)
                    n589 = local read "CRC16"() -> (w993:u16)
                    n590 = Concatenate Strings(w1000, "boot就绪查询..." ("字符串"), "\n") -> (w997:string)
                    n591 = Split Number(x=w993) -> (hi(x)=w991:u8, lo(x)=w992:u8)
                    n592 = local write "Info："(w997) -> ()
                    n593 = Bundle(cluster=w1004, "ID"=w1001, "TimeStamp"=u8 0 ("RemoteFlag"), "TimeFlag"=u8 1, "SendType"=u8 0 ("DataLen"), "RemoteFlag"=u8 0, "ExternFlag"=u8 1, "DataLen"=u8 8, u8 1 ("元素"), w990, w989, w988, w987, w991, w992, w1011, w1011, w1011) -> (w1008:T2)  [unwired: 1 in]
                    n594 = dll-call lib="F:/Bluewave New Energy/SVN_Work/BMS_BootLoader/trunk/BMS_Bootloader/AutoBurn/Settings/ControlCAN.dll" fn="VCI_Transmit"("DeviceType"=w1007, "DeviceInd"=w1006, "CANInd"=w1005, "pSend"=w1008, "Len"=u32 1) -> ()  [unwired: 5 in, 6 out]
                  }
                }
                n595 = local read "Info："() -> (w975:string)
                n596 = local write "进入烧录"(FALSE ("进入烧录")) -> ()
                n597 = Concatenate Strings(w975, "boot模式应答...成功" ("字符串"), "\n") -> (w978:string)
                n598 = local write "Info："(w978) -> ()
                "boot模式应答...成功" <- TRUE
              }
            }
          }
          frame 168192..168224, 168447 {
            n599 = To Unsigned Byte Integer(number=w1021) -> (unsigned 8bit integer=w1020:u8)
            n600 = Equal?(x=w1023, y=u8 85) -> (x = y?=w1019:bool)
            n601 = case shown="真" w1019 {
              tunnel: w1020 -> [_ w1043]
              frame False {
                n602 = flat-sequence {
                  frame #0 {
                    n603 = local read "设备索引"() -> (w1036:u32)
                    n604 = local read "CAN路数"() -> (w1034:u32)
                    n605 = local read "波特率"() -> (w1035:T1)
                    n606 = local read "滤波方式"() -> (w1033:u8)
                    n607 = local read "工作方式"() -> (w1032:u8)
                    n608 = local read "类型"() -> (w1037:u32)
                    n609 = call "CAN_Init.vi"("设备类型"=w1037, "设备索引"=w1036, "波特率"=w1035, "CAN路数"=w1034, "操作类型"=enum16{"初始化CAN", "关闭CAN"}."关闭CAN", "滤波方式"=w1033, "工作方式"=w1032) -> ()  [unwired: 11 in, 2 out]
                    n610 = Wait (ms)(milliseconds to wait=u32 2000 ("等待时间（毫秒）")) -> ()  [unwired: 1 out]
                  }
                  frame #1 {
                    n611 = Quit LabVIEW(quit? (T)=TRUE ("退出？(T)")) -> ()
                  }
                }
                n612 = local write "update flag"(FALSE ("update flag")) -> ()
                n613 = local read "Info："() -> (w1026:string)
                n614 = Concatenate Strings(w1026, "boot就绪应答...失败" ("字符串"), "\n") -> (w1029:string)
                n615 = One Button Dialog(message="程序下载错误，请断电重试！" ("消息")) -> ()  [unwired: 1 in, 1 out]
                n616 = local write "Info："(w1029) -> ()
              }
              frame True {
                n617 = stacked-sequence {
                  tunnel: w1043 -> [_ w1052]
                  frame #0 {
                    n618 = disable-structure shown="启用" {
                      frame Enabled {
                        n619 = local read "CAN路数"() -> (w1046:u32)
                        n620 = local read "设备索引"() -> (w1047:u32)
                        n621 = local read "类型"() -> (w1048:u32)
                        n622 = dll-call lib="F:/Bluewave New Energy/SVN_Work/BMS_BootLoader/trunk/BMS_Bootloader/AutoBurn/Settings/ControlCAN.dll" fn="VCI_ClearBuffer" label="VCI_Clearbuffer"(error in=errorcluster {"status"=FALSE, "code"=0, "source"=""} ("错误输入（无错误）"), "DeviceType"=w1048, "DeviceInd"=w1047, "CANInd"=w1046) -> (error out=→"错误输出 13":errorcluster)  [unwired: 3 in, 4 out]
                      }
                      frame Disabled {
                      }
                    }
                  }
                  frame #1 {
                    w1053 = u16 256 ("y")
                    w1068 = u8 0 ("元素")
                    n623 = local read "目标板类型"() -> (w1050:enum16{"BCU/主板", "BMU/从板"})
                    n624 = case shown="\"BCU/主板\", 默认" w1050 {
                      tunnel: [u16 0 ("请选择板号") w1075] -> w1049
                      frame "BCU/主板", Default {
                      }
                      frame "BMU/从板" {
                        n625 = local read "请选择板号"() -> (w1075:u16)
                      }
                    }
                    n626 = local read "设备索引"() -> (w1063:u32)
                    n627 = local read "CAN路数"() -> (w1062:u32)
                    n628 = local read "类型"() -> (w1064:u32)
                    n629 = local read "Info："() -> (w1054:string)
                    n630 = Multiply(x=w1049, y=w1053) -> ()  [unwired: 1 out]
                    n631 = Multiply(x=w1053, y=w1052) -> (x*y=w1051:u16)
                    n632 = Concatenate Strings(w1054, "boot擦除flash请求..." ("字符串"), "\n") -> (w1057:string)
                    n633 = Add(x=u32 196753 ("ID"), y=w1051) -> (x+y=w1058:u32)
                    n634 = local write "Info："(w1057) -> ()
                    n635 = local read "VCI_CAN_OBJ_T"() -> (w1061:T2)
                    n636 = Bundle(cluster=w1061, "ID"=w1058, "TimeStamp"=u8 0 ("RemoteFlag"), "TimeFlag"=u8 1, "SendType"=u8 0 ("DataLen"), "RemoteFlag"=u8 0, "ExternFlag"=u8 1, "DataLen"=u8 8, u8 1 ("元素"), w1068, w1068, w1068) -> (w1065:T2)  [unwired: 7 in]
                    n637 = dll-call lib="F:/Bluewave New Energy/SVN_Work/BMS_BootLoader/trunk/BMS_Bootloader/AutoBurn/Settings/ControlCAN.dll" fn="VCI_Transmit"("DeviceType"=w1064, "DeviceInd"=w1063, "CANInd"=w1062, "pSend"=w1065, "Len"=u32 1) -> ()  [unwired: 5 in, 6 out]
                  }
                }
                n638 = local read "Info："() -> (w1039:string)
                n639 = Concatenate Strings(w1039, "boot就绪应答...成功" ("字符串"), "\n") -> (w1042:string)
                n640 = local write "Info："(w1042) -> ()
              }
            }
          }
          frame 233728..233760, 233983 {
            n641 = To Unsigned Byte Integer(number=w1077) -> (unsigned 8bit integer=w1076:u8)
            n642 = Equal?(x=w1084, y=u8 85) -> (x = y?=w1082:bool)
            n643 = case shown="假" w1082 {
              tunnel: w1081 -> [_ w1115]
              tunnel: w1080 -> [_ w1114]
              tunnel: w1079 -> [_ w1113]
              tunnel: w1078 -> [_ w1112]
              tunnel: w1076 -> [_ w1109]
              frame False {
                n644 = local write "update flag"(FALSE ("update flag")) -> ()
                n645 = local read "Info："() -> (w1087:string)
                n646 = Concatenate Strings(w1087, "boot擦除flash应答...失败" ("字符串"), "\n") -> (w1090:string)
                n647 = local write "Info："(w1090) -> ()
                n648 = One Button Dialog(message="程序下载错误，请断电重试！" ("消息")) -> ()  [unwired: 1 in, 1 out]
                n649 = flat-sequence {
                  frame #0 {
                    n650 = local read "设备索引"() -> (w1097:u32)
                    n651 = local read "CAN路数"() -> (w1095:u32)
                    n652 = local read "波特率"() -> (w1096:T1)
                    n653 = local read "滤波方式"() -> (w1094:u8)
                    n654 = local read "工作方式"() -> (w1093:u8)
                    n655 = local read "类型"() -> (w1098:u32)
                    n656 = call "CAN_Init.vi"("设备类型"=w1098, "设备索引"=w1097, "波特率"=w1096, "CAN路数"=w1095, "操作类型"=enum16{"初始化CAN", "关闭CAN"}."关闭CAN", "滤波方式"=w1094, "工作方式"=w1093) -> ()  [unwired: 11 in, 2 out]
                    n657 = Wait (ms)(milliseconds to wait=u32 2000 ("等待时间（毫秒）")) -> ()  [unwired: 1 out]
                  }
                  frame #1 {
                    n658 = Quit LabVIEW(quit? (T)=TRUE ("退出？(T)")) -> ()
                  }
                }
              }
              frame True {
                w1110 = 0 ("索引")
                n659 = local read "子数组"() -> (w1111:string[])
                n660 = flat-sequence {
                  frame #0 {
                    n661 = local read "Info："() -> (w1120:string)
                    n662 = Concatenate Strings(w1120, "boot擦除flash应答...成功" ("字符串"), "\n") -> (w1122:string)
                    n663 = local write "Info："(w1122) -> ()
                  }
                  frame #1 {
                    n664 = local read "Info："() -> (w1127:string)
                    n665 = Concatenate Strings(w1127, "开始下载数据..." ("字符串"), "\n") -> (w1125:string)
                    n666 = Tick Count (ms)() -> (millisecond timer value=w1123:u32)
                    n667 = local write "Info："(w1125) -> ()
                    n668 = local write "开始下载数据"(w1123) -> ()
                    "开始下载数据" <- TRUE
                  }
                }
                n669 = Array Size(array=w1111) -> (size(s)=w1116:i32)
                n670 = Index Array(array=w1111, index=w1110) -> (element=w1100:string)
                n671 = String Subset(string=w1100, offset (0)=1 ("偏移量(0)"), length (rest)=1 ("长度（子字符串长度）")) -> (substring=w1105:string)
                n672 = case shown="\"2\"" w1105 {
                  tunnel: ["01" ("子字符串(\"\")") "02" ("子字符串(\"\")")] -> w1104
                  frame "1", Default {
                  }
                  frame "2" {
                  }
                }
                n673 = String Subset(string=w1100, offset (0)=2 ("偏移量(0)")) -> (substring=w1102:string)  [unwired: 1 in]
                n674 = Concatenate Strings("FFFFFFFFFFFF" ("子字符串(\"\")"), w1104, w1102) -> ()  [unwired: 1 out]
                n675 = while {
                  tunnel: w1115 -> [w1152]
                  tunnel: w1114 -> [w1151]
                  tunnel: w1113 -> [w1150]
                  tunnel: w1112 -> [w1149]
                  shift-right: [w1144] -> _
                  shift-left: w1100 -> [w1145]
                  tunnel: w1116 -> [w1142]
                  tunnel: w1110 -> [w1138]
                  tunnel: w1109 -> [w1132]
                  tunnel: u16 1 ("y") -> [w1131]
                  stop <- w1137 stop-if-true
                  w1135 = u16 256 ("y")
                  n676 = String Length(string=w1145) -> (length=w1143:i32)
                  n677 = Greater Or Equal?(x=w1143, y=16) -> (x >= y?=w1146:bool)
                  n678 = local read "目标板类型"() -> (w1130:enum16{"BCU/主板", "BMU/从板"})
                  n679 = case shown="\"BCU/主板\", 默认" w1130 {
                    tunnel: [u16 0 ("请选择板号") w1154] -> w1129
                    frame "BCU/主板", Default {
                    }
                    frame "BMU/从板" {
                      n680 = local read "请选择板号"() -> (w1154:u16)
                    }
                  }
                  n681 = Multiply(x=w1129, y=w1135) -> ()  [unwired: 1 out]
                  n682 = Multiply(x=w1135, y=w1132) -> (x*y=w1134:u16)
                  n683 = Divide(x=w1138, y=w1142) -> (x/y=w1141:dbl)
                  n684 = Add(x=u32 262289 ("ID"), y=w1134) -> (x+y=w1133:u32)
                  n685 = Multiply(x=w1141, y=100.0) -> (x*y=w1139:dbl)
                  n686 = case shown="假" w1146 {
                    tunnel: w1152 -> [w1183 w1195]
                    tunnel: w1151 -> [w1182 w1194]
                    tunnel: w1150 -> [w1181 w1193]
                    tunnel: w1149 -> [w1180 w1192]
                    tunnel: w1145 -> [w1156 w1191]
                    tunnel: [w1161 w1190] -> w1144
                    tunnel: [FALSE TRUE] -> w1137
                    tunnel: w1143 -> [_ w1188]
                    tunnel: w1143 -> [_ w1187]
                    tunnel: w1133 -> [w1159 w1186]
                    tunnel: w1131 -> [_ w1185]
                    frame True {
                      w1177 = u8 0 ("元素")
                      n687 = String Subset(string=w1156, length (rest)=16 ("长度（剩余）")) -> (substring=w1155:string)  [unwired: 1 in]
                      n688 = String Subset(string=w1156, offset (0)=16 ("偏移量(0)")) -> (substring=w1161:string)  [unwired: 1 in]
                      n689 = call "ASCII_To_Hex.vi"("ASCII String"=w1155) -> ("hex数组"=w1157:u16[])  [unwired: 6 in, 4 out]
                      n690 = Index Array(array=w1157) -> (element #1=w1169:u16, element #2=w1168:u16, element #3=w1167:u16, element #4=w1166:u16, element #5=w1165:u16, element #6=w1164:u16, element #7=w1163:u16, element #8=w1162:u16)  [unwired: 8 in]
                      n691 = Bundle(cluster=w1183, "ID"=w1159, "TimeStamp"=u8 0 ("RemoteFlag"), "TimeFlag"=u8 1, "SendType"=u8 0 ("DataLen"), "RemoteFlag"=u8 0, "ExternFlag"=u8 1, "DataLen"=u8 8, w1169, w1168, w1167, w1166, w1165, w1164, w1163, w1162, w1177, w1177, w1177) -> (w1172:T2)
                      n692 = dll-call lib="F:/Bluewave New Energy/SVN_Work/BMS_BootLoader/trunk/BMS_Bootloader/AutoBurn/Settings/ControlCAN.dll" fn="VCI_Transmit"("DeviceType"=w1182, "DeviceInd"=w1181, "CANInd"=w1180, "pSend"=w1172, "Len"=u32 1) -> ()  [unwired: 5 in, 6 out]
                    }
                    frame False {
                      n693 = Greater Than 0?(x=w1188) -> (x > 0?=w1184:bool)
                      n694 = case shown="真" w1184 {
                        tunnel: w1195 -> [w1226 w1236]
                        tunnel: w1194 -> [w1225 w1235]
                        tunnel: w1193 -> [w1224 w1234]
                        tunnel: w1192 -> [w1223 w1233]
                        tunnel: w1191 -> [w1213 _]
                        tunnel: [w1204 _] -> w1190
                        tunnel: w1187 -> [_ w1231]
                        tunnel: w1186 -> [w1200 w1230]
                        tunnel: w1185 -> [_ w1229]
                        tunnel: w1185 -> [w1199 _]
                        frame True {
                          w1220 = u8 0 ("元素")
                          n695 = Wait (ms)(milliseconds to wait=u32 20 ("等待时间（毫秒）")) -> ()  [unwired: 1 out]
                          n696 = String Subset(string=w1213, offset (0)=16 ("偏移量(0)")) -> (substring=w1204:string)  [unwired: 1 in]
                          n697 = String Subset(string=w1213, length (rest)=16 ("长度（剩余）")) -> (substring=w1197:string)  [unwired: 1 in]
                          n698 = call "ASCII_To_Hex.vi"("ASCII String"=w1197) -> ("hex数组"=w1196:u16[])  [unwired: 6 in, 4 out]
                          n699 = Index Array(array=w1196) -> (element #1=w1212:u16, element #2=w1211:u16, element #3=w1210:u16, element #4=w1209:u16, element #5=w1208:u16, element #6=w1207:u16, element #7=w1206:u16, element #8=w1205:u16)  [unwired: 8 in]
                          n700 = Bundle(cluster=w1226, "ID"=w1200, "TimeStamp"=u8 0 ("RemoteFlag"), "TimeFlag"=u8 1, "SendType"=u8 0 ("DataLen"), "RemoteFlag"=u8 0, "ExternFlag"=w1199, "DataLen"=u8 8, w1212, w1211, w1210, w1209, w1208, w1207, w1206, w1205, w1220, w1220, w1220) -> (w1215:T2)
                          n701 = dll-call lib="F:/Bluewave New Energy/SVN_Work/BMS_BootLoader/trunk/BMS_Bootloader/AutoBurn/Settings/ControlCAN.dll" fn="VCI_Transmit"(error in="错误输入（无错误） 3", "DeviceType"=w1225, "DeviceInd"=w1224, "CANInd"=w1223, "pSend"=w1215, "Len"=u32 1) -> (error out=→"错误输出 14":errorcluster)  [unwired: 4 in, 5 out]
                        }
                        frame False {
                          (unwired) TRUE
                          n702 = Quotient & Remainder(x=w1231, y=8) -> ()  [unwired: 2 out]
                          n703 = Wait (ms)(milliseconds to wait=u32 20 ("等待时间（毫秒）")) -> ()  [unwired: 1 out]
                          n704 = case shown="0" 1 {
                            tunnel: w1236 -> [w1261 _]
                            tunnel: w1235 -> [w1260 _]
                            tunnel: w1234 -> [w1259 _]
                            tunnel: w1233 -> [w1258 _]
                            tunnel: w1230 -> [w1238 _]
                            tunnel: w1229 -> [w1237 _]
                            frame 0 {
                              w1255 = u8 0 ("元素")
                              n705 = Index Array(array=u8[] [0, 0, 0, 0, 0, 0, 0, 0] ("数组")) -> (element #1=w1249:u8, element #2=w1248:u8, element #3=w1247:u8, element #4=w1246:u8, element #5=w1245:u8, element #6=w1244:u8, element #7=w1243:u8, element #8=w1242:u8)  [unwired: 8 in]
                              n706 = Bundle(cluster=w1261, "ID"=w1238, "TimeStamp"=u8 0 ("RemoteFlag"), "TimeFlag"=u8 1, "SendType"=u8 0 ("DataLen"), "RemoteFlag"=u8 0, "ExternFlag"=w1237, "DataLen"=u8 8, w1249, w1248, w1247, w1246, w1245, w1244, w1243, w1242, w1255, w1255, w1255) -> (w1250:T2)
                              n707 = dll-call lib="F:/Bluewave New Energy/SVN_Work/BMS_BootLoader/trunk/BMS_Bootloader/AutoBurn/Settings/ControlCAN.dll" fn="VCI_Transmit"(error in="错误输入（无错误） 4", "DeviceType"=w1260, "DeviceInd"=w1259, "CANInd"=w1258, "pSend"=w1250, "Len"=u32 1) -> (error out=→"错误输出 15":errorcluster)  [unwired: 4 in, 5 out]
                            }
                            frame 1, Default {
                            }
                          }
                        }
                      }
                    }
                  }
                  n708 = local write "进度"(w1139) -> ()
                  n709 = Wait (ms)(milliseconds to wait=u32 5 ("等待时间（毫秒）")) -> ()  [unwired: 1 out]
                }
                "当前发送行" <- w1110
              }
            }
          }
          frame 299264..299296, 299519 {
            n710 = To Unsigned Byte Integer(number=w1265) -> (unsigned 8bit integer=w1264:u8)
            n711 = Equal?(x=w1263, y=u8 85) -> (x = y?=w1262:bool)
            n712 = case shown="假" w1262 {
              tunnel: w1269 -> [_ w1295]
              tunnel: w1268 -> [_ w1294]
              tunnel: w1267 -> [_ w1293]
              tunnel: w1266 -> [_ w1292]
              tunnel: w1264 -> [_ w1286]
              frame False {
                n713 = local write "update flag"(FALSE ("update flag")) -> ()
                n714 = local read "Info："() -> (w1273:string)
                n715 = Concatenate Strings(w1273, "扇区数据传输应答...失败" ("字符串"), "\n") -> (w1276:string)
                n716 = One Button Dialog(message="程序下载错误，请断电重试！" ("消息")) -> ()  [unwired: 1 in, 1 out]
                n717 = local write "Info："(w1276) -> ()
              }
              frame True {
                n718 = local read "当前发送行"() -> (w1290:i32)
                n719 = local read "子数组"() -> (w1291:string[])
                n720 = Array Size(array=w1291) -> (size(s)=w1296:i32)
                n721 = Increment(x=w1290) -> (x+1=w1289:i32)
                n722 = Index Array(array=w1291, index=w1289) -> (element=w1278:string)
                n723 = String Subset(string=w1278, offset (0)=1 ("偏移量(0)"), length (rest)=1 ("长度（子字符串长度）")) -> (substring=w1283:string)
                n724 = case shown="\"2\"" w1283 {
                  tunnel: ["01" ("子字符串(\"\")") "02" ("子字符串(\"\")")] -> w1281
                  frame "1", Default {
                  }
                  frame "2" {
                  }
                }
                n725 = Tick Count (ms)() -> (millisecond timer value=w1277:u32)
                n726 = local write "当前发送行"(w1289) -> ()
                n727 = String Subset(string=w1278, offset (0)=2 ("偏移量(0)")) -> (substring=w1279:string)  [unwired: 1 in]
                n728 = String Length(string=w1278) -> (length=w1288:i32)
                n729 = local write "开始下载数据"(w1277) -> ()
                n730 = Concatenate Strings("FFFFFFFFFFFF" ("子字符串(\"\")"), w1281, w1279) -> ()  [unwired: 1 out]
                n731 = Greater Than 0?(x=w1288) -> (x > 0?=w1287:bool)
                n732 = case shown="假" w1287 {
                  tunnel: w1296 -> [_ w1361]
                  tunnel: w1295 -> [w1340 w1360]
                  tunnel: w1294 -> [w1339 w1359]
                  tunnel: w1293 -> [w1338 w1358]
                  tunnel: w1292 -> [w1337 w1357]
                  tunnel: w1289 -> [_ w1356]
                  tunnel: w1278 -> [_ w1355]
                  tunnel: w1286 -> [w1310 w1350]
                  frame False {
                    w1301 = "BURNRESULT" ("section")
                    w1334 = u8 0 ("元素")
                    n733 = Multiply(x=w1310, y=u16 256) -> (x*y=w1307:u16)
                    n734 = local write "update flag"(FALSE ("update flag")) -> ()
                    n735 = local write "开始下载数据"(FALSE ("开始下载数据")) -> ()
                    n736 = Add(x=u32 327825 ("ID"), y=w1307) -> (x+y=w1308:u32)
                    n737 = String To Byte Array(string="" ("字符串")) -> (unsigned byte array=w1328:u8[])
                    n738 = flat-sequence {
                      frame #0 {
                        n739 = local read "设备索引"() -> (w1347:u32)
                        n740 = local read "CAN路数"() -> (w1345:u32)
                        n741 = local read "波特率"() -> (w1346:T1)
                        n742 = local read "滤波方式"() -> (w1344:u8)
                        n743 = local read "工作方式"() -> (w1343:u8)
                        n744 = local read "类型"() -> (w1348:u32)
                        n745 = call "CAN_Init.vi"("设备类型"=w1348, "设备索引"=w1347, "波特率"=w1346, "CAN路数"=w1345, "操作类型"=enum16{"初始化CAN", "关闭CAN"}."关闭CAN", "滤波方式"=w1344, "工作方式"=w1343) -> ()  [unwired: 11 in, 2 out]
                        n746 = Wait (ms)(milliseconds to wait=u32 2000 ("等待时间（毫秒）")) -> ()  [unwired: 1 out]
                      }
                      frame #1 {
                        n747 = Quit LabVIEW(quit? (T)=TRUE ("退出？(T)")) -> ()
                      }
                    }
                    n748 = Index Array(array=w1328) -> (element #1=w1327:u8, element #2=w1326:u8, element #3=w1325:u8, element #4=w1324:u8, element #5=w1323:u8, element #6=w1322:u8, element #7=w1321:u8, element #8=w1320:u8)  [unwired: 8 in]
                    n749 = Bundle(cluster=w1340, "ID"=w1308, "TimeStamp"=u8 0 ("RemoteFlag"), "TimeFlag"=u8 1, "SendType"=u8 0 ("DataLen"), "RemoteFlag"=u8 0, "ExternFlag"=u8 1, "DataLen"=u8 8, w1327, w1326, w1325, w1324, w1323, w1322, w1321, w1320, w1334, w1334, w1334) -> (w1329:T2)
                    n750 = dll-call lib="F:/Bluewave New Energy/SVN_Work/BMS_BootLoader/trunk/BMS_Bootloader/AutoBurn/Settings/ControlCAN.dll" fn="VCI_Transmit"(error in="错误输入（无错误） 7", "DeviceType"=w1339, "DeviceInd"=w1338, "CANInd"=w1337, "pSend"=w1329, "Len"=u32 1) -> (error out=→"错误输出 18":errorcluster)  [unwired: 4 in, 5 out]
                    n751 = local read "Info："() -> (w1313:string)
                    n752 = call <vilib>:"Open Config Data.vi"("configuration file path"=path "D:/BlueWay/configresult.ini") -> ("refnum"=w1300:T4)  [unwired: 8 in, 2 out]
                    n753 = Concatenate Strings(w1313, "应用刷写完成..请重新上电！" ("字符串"), "\n") -> (w1316:string)
                    n754 = local write "Info："(w1316) -> ()
                    n755 = call-poly <vilib>:"Write Key.vi"("section"=w1301, "value"="PASS" ("section"), "key"=w1301, "refnum"=w1300) -> ("error out"=w1304:errorcluster, "refnum out"=w1303:T4)  [unwired: 5 in, 1 out]
                    n756 = call <vilib>:"Close Config Data.vi"("error in (no error)"=w1304, "refnum"=w1303) -> ()  [unwired: 8 in, 2 out]
                  }
                  frame True {
                    n757 = Multiply(x=w1350, y=u16 256) -> (x*y=w1353:u16)
                    n758 = Add(x=u32 262289 ("ID"), y=w1353) -> (x+y=w1351:u32)
                    n759 = while {
                      tunnel: w1360 -> [w1377]
                      tunnel: w1359 -> [w1376]
                      tunnel: w1358 -> [w1375]
                      tunnel: w1357 -> [w1374]
                      shift-right: [w1370] -> _
                      shift-left: w1355 -> [w1371]
                      tunnel: w1361 -> [w1368]
                      tunnel: w1356 -> [w1364]
                      tunnel: w1351 -> [w1362]
                      stop <- w1363 stop-if-true
                      n760 = String Length(string=w1371) -> (length=w1369:i32)
                      n761 = Greater Or Equal?(x=w1369, y=16) -> (x >= y?=w1372:bool)
                      n762 = case shown="真" w1372 {
                        tunnel: w1377 -> [w1406 w1418]
                        tunnel: w1376 -> [w1405 w1417]
                        tunnel: w1375 -> [w1404 w1416]
                        tunnel: w1374 -> [w1403 w1415]
                        tunnel: w1371 -> [w1393 w1414]
                        tunnel: [w1383 w1413] -> w1370
                        tunnel: [FALSE TRUE] -> w1363
                        tunnel: w1369 -> [_ w1411]
                        tunnel: w1369 -> [_ w1410]
                        tunnel: w1362 -> [w1381 w1408]
                        frame True {
                          (unwired) u8 1 ("ExternFlag")
                          w1400 = u8 0 ("元素")
                          n763 = String Subset(string=w1393, offset (0)=16 ("偏移量(0)")) -> (substring=w1383:string)  [unwired: 1 in]
                          n764 = String Subset(string=w1393, length (rest)=16 ("长度（剩余）")) -> (substring=w1379:string)  [unwired: 1 in]
                          n765 = call "ASCII_To_Hex.vi"("ASCII String"=w1379) -> ("hex数组"=w1378:u16[])  [unwired: 6 in, 4 out]
                          n766 = Index Array(array=w1378) -> (element #1=w1391:u16, element #2=w1390:u16, element #3=w1389:u16, element #4=w1388:u16, element #5=w1387:u16, element #6=w1386:u16, element #7=w1385:u16, element #8=w1384:u16)  [unwired: 8 in]
                          n767 = Bundle(cluster=w1406, "ID"=w1381, "TimeStamp"=u8 0 ("RemoteFlag"), "TimeFlag"=u8 1, "SendType"=u8 0 ("DataLen"), "RemoteFlag"=u8 0, "ExternFlag"=u8 1, "DataLen"=u8 8, w1391, w1390, w1389, w1388, w1387, w1386, w1385, w1384, w1400, w1400, w1400) -> (w1395:T2)
                          n768 = dll-call lib="F:/Bluewave New Energy/SVN_Work/BMS_BootLoader/trunk/BMS_Bootloader/AutoBurn/Settings/ControlCAN.dll" fn="VCI_Transmit"("DeviceType"=w1405, "DeviceInd"=w1404, "CANInd"=w1403, "pSend"=w1395, "Len"=u32 1) -> ()  [unwired: 5 in, 6 out]
                        }
                        frame False {
                          n769 = Greater Than 0?(x=w1411) -> ()  [unwired: 1 out]
                          n770 = case shown="真" TRUE {
                            tunnel: w1418 -> [w1449 w1456]
                            tunnel: w1417 -> [w1448 w1455]
                            tunnel: w1416 -> [w1447 w1454]
                            tunnel: w1415 -> [w1446 w1453]
                            tunnel: w1414 -> [w1436 _]
                            tunnel: [w1427 _] -> w1413
                            tunnel: w1410 -> [_ w1451]
                            tunnel: w1408 -> [w1424 _]
                            tunnel: [w1422 _] -> w1407
                            frame True {
                              w1443 = u8 0 ("元素")
                              n771 = String Subset(string=w1436, length (rest)=16 ("长度（剩余）")) -> (substring=w1421:string)  [unwired: 1 in]
                              n772 = String Subset(string=w1436, offset (0)=16 ("偏移量(0)")) -> (substring=w1427:string)  [unwired: 1 in]
                              n773 = call "ASCII_To_Hex.vi"("ASCII String"=w1421) -> ("hex数组"=w1420:u16[])  [unwired: 6 in, 4 out]
                              n774 = Index Array(array=w1420) -> (element #1=w1435:u16, element #2=w1434:u16, element #3=w1433:u16, element #4=w1432:u16, element #5=w1431:u16, element #6=w1430:u16, element #7=w1429:u16, element #8=w1428:u16)  [unwired: 8 in]
                              n775 = Bundle(cluster=w1449, "ID"=w1424, "TimeStamp"=u8 0 ("RemoteFlag"), "TimeFlag"=u8 1, "SendType"=u8 0 ("DataLen"), "RemoteFlag"=u8 0, "ExternFlag"=u8 1, "DataLen"=u8 8, w1435, w1434, w1433, w1432, w1431, w1430, w1429, w1428, w1443, w1443, w1443) -> (w1438:T2)
                              n776 = dll-call lib="F:/Bluewave New Energy/SVN_Work/BMS_BootLoader/trunk/BMS_Bootloader/AutoBurn/Settings/ControlCAN.dll" fn="VCI_Transmit"(error in="错误输入（无错误） 5", "DeviceType"=w1448, "DeviceInd"=w1447, "CANInd"=w1446, "pSend"=w1438, "Len"=u32 1) -> (error out=w1422:errorcluster)  [unwired: 4 in, 5 out]
                              "错误输出 16" <- w1422
                            }
                            frame False {
                              n777 = Quotient & Remainder(x=w1451, y=8) -> (x-y*floor(x/y)=w1450:i32)  [unwired: 1 out]
                              n778 = case shown="0" w1450 {
                                tunnel: w1456 -> [w1480 _]
                                tunnel: w1455 -> [w1479 _]
                                tunnel: w1454 -> [w1478 _]
                                tunnel: w1453 -> [w1477 _]
                                frame 0 {
                                w1473 = u8 0 ("元素")
                                n779 = Index Array(array=u8[] [0, 0, 0, 0, 0, 0, 0, 0] ("数组")) -> (element #1=w1467:u8, element #2=w1466:u8, element #3=w1465:u8, element #4=w1464:u8, element #5=w1463:u8, element #6=w1462:u8, element #7=w1461:u8, element #8=w1460:u8)  [unwired: 8 in]
                                n780 = Bundle(cluster=w1480, "ID"=u32 5, "TimeStamp"=u8 0 ("RemoteFlag"), "TimeFlag"=u8 1, "SendType"=u8 0 ("DataLen"), "RemoteFlag"=u8 0, "DataLen"=u8 8, w1467, w1466, w1465, w1464, w1463, w1462, w1461, w1460, w1473, w1473, w1473) -> (w1468:T2)  [unwired: 1 in]
                                n781 = dll-call lib="F:/Bluewave New Energy/SVN_Work/BMS_BootLoader/trunk/BMS_Bootloader/AutoBurn/Settings/ControlCAN.dll" fn="VCI_Transmit"(error in="错误输入（无错误） 6", "DeviceType"=w1479, "DeviceInd"=w1478, "CANInd"=w1477, "pSend"=w1468, "Len"=u32 1) -> (error out=→"错误输出 17":errorcluster)  [unwired: 4 in, 5 out]
                                }
                                frame 1, Default {
                                }
                              }
                            }
                          }
                          n782 = flat-sequence {
                            tunnel: w1407 -> [_]
                            frame #0 {
                              n783 = Wait (ms)(milliseconds to wait=u32 1 ("等待时间（毫秒）")) -> ()  [unwired: 1 out]
                            }
                          }
                        }
                      }
                      n784 = Divide(x=w1364, y=w1368) -> (x/y=w1367:dbl)
                      n785 = Multiply(x=w1367, y=100.0) -> (x*y=w1365:dbl)
                      n786 = local write "进度"(w1365) -> ()
                    }
                  }
                }
              }
            }
          }
          frame 254 {
            (unwired) TRUE
            n787 = disable-structure shown="禁用" {
              disable-tunnel: w1487 -> [w1497 _]
              disable-tunnel: w1486 -> [w1496 _]
              disable-tunnel: w1485 -> [w1495 _]
              disable-tunnel: w1484 -> [w1494 _]
              disable-tunnel: w1481 -> [w1490 _]
              frame Disabled {
                w1493 = FALSE ("进入烧录模式")
                n788 = Two Button Dialog(message="进入烧录模式!，是否开始烧录？\n如果BMS重新上电，请点取消！！" ("消息")) -> (T button?=w1488:bool)  [unwired: 2 in]
                n789 = case shown="真" w1488 {
                  tunnel: w1497 -> [w1503 w1530]
                  tunnel: w1496 -> [w1502 w1525]
                  tunnel: w1495 -> [w1501 w1524]
                  tunnel: w1494 -> [w1500 w1523]
                  tunnel: w1490 -> [w1498 w1526]
                  frame True {
                    n790 = stacked-sequence {
                      tunnel: w1503 -> [_ w1511]
                      tunnel: w1502 -> [w1506 w1510]
                      tunnel: w1501 -> [w1505 w1509]
                      tunnel: w1500 -> [w1504 w1508]
                      tunnel: w1498 -> [w1507 _]
                      frame #0 {
                        n791 = Flush Queue(queue=w1507) -> ()  [unwired: 1 in, 3 out]
                        n792 = dll-call lib="F:/Bluewave New Energy/SVN_Work/BMS_BootLoader/trunk/BMS_Bootloader/AutoBurn/Settings/ControlCAN.dll" fn="VCI_ClearBuffer" label="VCI_Clearbuffer"("DeviceType"=w1506, "DeviceInd"=w1505, "CANInd"=w1504) -> ()  [unwired: 4 in, 5 out]
                      }
                      frame #1 {
                        w1518 = u8 0 ("元素")
                        n793 = Bundle(cluster=w1511, "ID"=u32 0, "TimeStamp"=u8 0 ("RemoteFlag"), "TimeFlag"=u8 1, "SendType"=u8 0 ("DataLen"), "RemoteFlag"=u8 0, "ExternFlag"=u8 0, "DataLen"=u8 1, u8 2 ("元素"), w1518, w1518, w1518) -> (w1522:T2)  [unwired: 7 in]
                        n794 = dll-call lib="F:/Bluewave New Energy/SVN_Work/BMS_BootLoader/trunk/BMS_Bootloader/AutoBurn/Settings/ControlCAN.dll" fn="VCI_Transmit"("DeviceType"=w1510, "DeviceInd"=w1509, "CANInd"=w1508, "pSend"=w1522, "Len"=u32 1) -> ()  [unwired: 5 in, 6 out]
                      }
                    }
                    "进入烧录模式" <- TRUE ("进入烧录模式")
                  }
                  frame False {
                    n795 = Flush Queue(queue=w1526) -> (error out=w1528:errorcluster)  [unwired: 1 in, 2 out]
                    n796 = invoke on="Monitor" class="Bool" method="Reinit To Default"() -> ()  [unwired: 3 in, 3 out]
                    n797 = local write "Monitor_flag"(FALSE ("Monitor_flag")) -> ()
                    n798 = dll-call lib="F:/Bluewave New Energy/SVN_Work/BMS_BootLoader/trunk/BMS_Bootloader/AutoBurn/Settings/ControlCAN.dll" fn="VCI_ClearBuffer" label="VCI_Clearbuffer"(error in=w1528, "DeviceType"=w1525, "DeviceInd"=w1524, "CANInd"=w1523) -> (error out=w1527:errorcluster)  [unwired: 3 in, 4 out]
                    n799 = disable-structure shown="禁用" {
                      disable-tunnel: w1530 -> [w1535 _]
                      disable-tunnel: w1527 -> [w1534 _]
                      disable-tunnel: w1525 -> [w1533 _]
                      disable-tunnel: w1524 -> [w1532 _]
                      disable-tunnel: w1523 -> [w1531 _]
                      frame Disabled {
                        w1542 = u8 0 ("元素")
                        n800 = Bundle(cluster=w1535, "ID"=u32 0, "TimeStamp"=u8 0 ("RemoteFlag"), "TimeFlag"=u8 1, "SendType"=u8 0 ("DataLen"), "RemoteFlag"=u8 0, "ExternFlag"=u8 0, "DataLen"=u8 1, u8 5 ("元素"), w1542, w1542, w1542) -> (w1546:T2)  [unwired: 7 in]
                        n801 = dll-call lib="F:/Bluewave New Energy/SVN_Work/BMS_BootLoader/trunk/BMS_Bootloader/AutoBurn/Settings/ControlCAN.dll" fn="VCI_Transmit"(error in=w1534, "DeviceType"=w1533, "DeviceInd"=w1532, "CANInd"=w1531, "pSend"=w1546, "Len"=u32 1) -> ()  [unwired: 4 in, 6 out]
                      }
                      frame Enabled {
                      }
                    }
                  }
                }
                n802 = property on="烧录结果" class="Bool (严格)"("Colors [4]"=cluster{u32, u32}[] [{0, 0}] ("颜色[4]"), "BoolText.Text"="" ("布尔文本.文本")) -> ()  [unwired: 2 in, 2 out]
                n803 = local write "擦除完成"(w1493) -> ()
                n804 = local write "烧录结果"(w1493) -> ()
              }
              frame Enabled {
              }
            }
          }
          frame 253 {
            n805 = disable-structure shown="禁用" {
              disable-tunnel: w1556 -> [w1566 _]
              disable-tunnel: [w1565 _] -> w1555
              disable-tunnel: w1554 -> [w1564 _]
              disable-tunnel: w1553 -> [w1563 _]
              disable-tunnel: w1552 -> [w1562 _]
              disable-tunnel: w1551 -> [w1561 _]
              disable-tunnel: w1550 -> [w1560 _]
              disable-tunnel: [w1559 _] -> w1549
              disable-tunnel: w1548 -> [w1558 _]
              disable-tunnel: w1547 -> [w1557 _]
              frame Disabled {
                n806 = stacked-sequence {
                  tunnel: w1566 -> [_ w1584]
                  tunnel: [_ w1583] -> w1565
                  tunnel: w1564 -> [w1571 w1582]
                  tunnel: w1563 -> [w1570 w1581]
                  tunnel: w1562 -> [_ w1580]
                  tunnel: w1561 -> [w1569 w1579]
                  tunnel: w1560 -> [_ w1578]
                  tunnel: [_ w1577] -> w1559
                  tunnel: w1558 -> [_ w1576]
                  tunnel: w1557 -> [w1568 w1572]
                  frame #0 {
                    n807 = dll-call lib="F:/Bluewave New Energy/SVN_Work/BMS_BootLoader/trunk/BMS_Bootloader/AutoBurn/Settings/ControlCAN.dll" fn="VCI_ClearBuffer" label="VCI_Clearbuffer"("DeviceType"=w1571, "DeviceInd"=w1570, "CANInd"=w1569) -> ()  [unwired: 4 in, 5 out]
                    n808 = Flush Queue(queue=w1568) -> ()  [unwired: 1 in, 3 out]
                  }
                  frame #1 {
                    # "FD"
                    n809 = local read "子数组"() -> (w1586:string[])
                    n810 = while {
                      tunnel: w1586 -> [w1657] mode=indexing
                      tunnel: [w1653] -> w1585
                      tunnel: [w1649] -> w1575
                      i -> [w1653]
                      stop <- w1650 stop-if-true
                      n811 = Search/Split String(string=w1657, search string/char (-)="S9" ("搜索字符串/字符(-)")) -> (offset of match=w1655:i32)  [unwired: 1 in, 2 out]
                      n812 = Equal?(x=5000, y=w1653) -> (x = y?=w1651:bool)
                      n813 = Not Equal?(x=w1655, y=-1) -> (x != y?=w1649:bool)
                      n814 = Or(x=w1649, y=w1651) -> (x .or. y?=w1650:bool)
                    }
                    n815 = while {
                      tunnel: w1586 -> [w1666] mode=indexing
                      tunnel: [w1659] -> w1573
                      tunnel: [w1658] -> w1574
                      i -> [w1659]
                      stop <- w1661 stop-if-true
                      n816 = Equal?(x=5000, y=w1659) -> (x = y?=w1660:bool)
                      n817 = Search/Split String(string=w1666, search string/char (-)="S0" ("搜索字符串/字符(-)")) -> (offset of match=w1664:i32)  [unwired: 1 in, 2 out]
                      n818 = Not Equal?(x=w1664, y=-1) -> (x != y?=w1658:bool)
                      n819 = Or(x=w1658, y=w1660) -> (x .or. y?=w1661:bool)
                    }
                    n820 = case shown="真" w1575 {
                      tunnel: w1586 -> [_ w1632]
                      tunnel: w1585 -> [_ w1631]
                      tunnel: w1584 -> [w1588 _]
                      tunnel: [w1588 w1598] -> w1583
                      tunnel: w1582 -> [_ w1630]
                      tunnel: w1581 -> [_ w1629]
                      tunnel: w1580 -> [_ _]
                      tunnel: w1579 -> [_ w1628]
                      tunnel: w1578 -> [w1587 w1613]
                      tunnel: [w1587 w1611] -> w1577
                      tunnel: w1576 -> [_ w1595]
                      tunnel: w1574 -> [_ w1594]
                      tunnel: w1573 -> [_ w1593]
                      tunnel: w1572 -> [_ w1589]
                      frame False {
                      }
                      frame True {
                        n821 = case shown="真" w1594 {
                          tunnel: w1593 -> [_ w1635]
                          tunnel: [0 w1636] -> w1592
                          tunnel: [-1 w1635] -> w1591
                          frame False {
                          }
                          frame True {
                            n822 = Increment(x=w1635) -> (x+1=w1636:i32)
                          }
                        }
                        n823 = Subtract(x=w1631, y=w1591) -> (x-y=w1605:i32)
                        n824 = Decrement(x=w1605) -> (x-1=w1604:i32)
                        n825 = Array Subset(array=w1632, index=w1592, length=w1604) -> (w1602:string[])
                        n826 = Index Array(array=w1602, index=0 ("索引")) -> (element=w1610:string)
                        n827 = Delete From Array(array=w1602, length=1 ("长度"), index=0 ("索引")) -> (array with subset deleted=w1598:string[])  [unwired: 1 out]
                        n828 = String Subset(string=w1610, offset (0)=0 ("偏移量(0)"), length (rest)=2 ("长度（剩余）")) -> (substring=w1620:string)
                        n829 = String Subset(string=w1610, offset (0)=2 ("偏移量(0)"), length (rest)=2 ("长度（剩余）")) -> (substring=w1623:string)
                        n830 = Hexadecimal String To Number(string=w1623) -> (number=w1618:u32)  [unwired: 2 in, 1 out]
                        n831 = case shown="\"S2\"" w1620 {
                          tunnel: [4 ("偏移量(0)") 6 ("偏移量(0)")] -> w1609
                          tunnel: w1618 -> [w1641 w1647]
                          tunnel: [w1639 w1645] -> w1617
                          tunnel: [8 ("y") 10 ("y")] -> w1614
                          tunnel: ["S1" "S2"] -> w1606
                          frame "S1", Default {
                            n832 = Subtract(x=w1641, y=3) -> (x-y=w1639:u32)
                          }
                          frame "S2" {
                            n833 = Subtract(x=w1647, y=4) -> (x-y=w1645:u32)
                          }
                        }
                        "地址长度" <- w1609
                        n834 = Array Size(array=w1598) -> (size(s)=w1599:i32)
                        "大小" <- w1599
                        n835 = Divide(x=0, y=w1599) -> (x/y=w1596:dbl)
                        n836 = local write "进度"(w1596) -> ()
                        n837 = String Subset(string=w1610, offset (0)=4 ("偏移量(0)"), length (rest)=w1609) -> ()  [unwired: 1 out]
                        n838 = Multiply(x=u32 2, y=w1617) -> (x*y=w1615:u32)
                        "数据长度" <- w1615
                        n839 = String Subset(string=w1610, offset (0)=4 ("偏移量(0)"), length (rest)=w1609) -> (substring=w1607:string)
                        n840 = call "CAN R&W.vi"("设备类型"=w1630, "设备索引"=w1629, "CAN路数"=w1628, "DataLen"=u8 8, "写地址/数据"=enum16{"写地址", "写数据"}."写地址", "Data Input"=w1607, "枚举"=w1595, "TYPE"=w1606, "queue out"=w1589) -> ("发送的数据"=→"发送的数据":i32[])  [unwired: 17 in, 1 out]
                        n841 = String Subset(string=w1610, offset (0)=w1614, length (rest)=w1615) -> (substring=w1612:string)
                        n842 = Concatenate Strings(w1613, w1612) -> (w1611:string)
                      }
                    }
                  }
                }
                "擦除完成" <- TRUE ("擦写状态")
              }
              frame Enabled {
              }
            }
          }
          frame 252 {
            n843 = Unbundle(w1668) -> (w1669:u8, w1670:u8, w1671:u8, w1672:u8, w1673:u8, w1674:u8, w1675:u8, w1676:u8)  [unwired: 10 out]
            n844 = Build Array(w1669, w1670, w1671, w1672, w1673, w1674, w1675, w1676) -> (w1667:u8[])
            n845 = disable-structure shown="禁用" {
              disable-tunnel: w1684 -> [w1693 _]
              disable-tunnel: [w1692 _] -> w1683
              disable-tunnel: w1682 -> [w1691 _]
              disable-tunnel: w1681 -> [w1690 _]
              disable-tunnel: w1680 -> [w1689 _]
              disable-tunnel: w1679 -> [w1688 _]
              disable-tunnel: w1678 -> [w1687 _]
              disable-tunnel: w1677 -> [w1686 _]
              disable-tunnel: w1667 -> [w1685 _]
              frame Disabled {
                n846 = stacked-sequence {
                  tunnel: w1693 -> [_ w1716]
                  tunnel: [_ w1715] -> w1692
                  tunnel: w1691 -> [w1697 w1714]
                  tunnel: w1690 -> [w1696 w1713]
                  tunnel: w1689 -> [w1695 w1712]
                  tunnel: w1688 -> [_ w1710]
                  tunnel: w1687 -> [_ w1709]
                  tunnel: w1685 -> [_ w1703]
                  tunnel: w1686 -> [w1694 w1698]
                  frame #0 {
                    n847 = dll-call lib="F:/Bluewave New Energy/SVN_Work/BMS_BootLoader/trunk/BMS_Bootloader/AutoBurn/Settings/ControlCAN.dll" fn="VCI_ClearBuffer" label="VCI_Clearbuffer"("DeviceType"=w1697, "DeviceInd"=w1696, "CANInd"=w1695) -> ()  [unwired: 4 in, 5 out]
                    n848 = Flush Queue(queue=w1694) -> ()  [unwired: 1 in, 3 out]
                  }
                  frame #1 {
                    # "FC"
                    n849 = local read "发送的数据"() -> (w1708:i32[])
                    n850 = String Length(string=w1716) -> (length=w1717:i32)
                    n851 = Array Subset(array=w1703, index=1 ("索引"), length=6 ("长度")) -> (w1701:u8[])
                    n852 = Array Size(array=w1710) -> (size(s)=w1711:i32)
                    n853 = Array Subset(array=w1708, index=1 ("索引"), length=6 ("长度")) -> (w1702:i32[])
                    n854 = Greater Than 0?(x=w1717) -> (x > 0?=w1718:bool)
                    n855 = Equal?(x=w1702, y=w1701) -> (x = y?=w1700:bool[])
                    n856 = And Array Elements(Boolean array=w1700) -> (logical AND=w1699:bool)
                    n857 = case shown="假" w1699 {
                      tunnel: w1718 -> [_ w1730]
                      tunnel: w1717 -> [_ w1729]
                      tunnel: w1716 -> [_ w1728]
                      tunnel: [_ w1727] -> w1715
                      tunnel: w1714 -> [_ w1726]
                      tunnel: w1713 -> [_ w1725]
                      tunnel: w1712 -> [_ w1724]
                      tunnel: w1711 -> [_ w1723]
                      tunnel: w1709 -> [_ w1722]
                      tunnel: w1698 -> [_ w1721]
                      frame False {
                        w1719 = "失败" ("布尔文本.文本")
                        w1720 = cluster{u32, u32}[] [{16711680, 0}] ("颜色[4]")
                        n858 = property on="校验" class="Bool (严格)"("Colors [4]"=w1720, "BoolText.Text"=w1719) -> ()  [unwired: 2 in, 2 out]
                        n859 = property on="烧录结果" class="Bool (严格)"("Colors [4]"=w1720, "BoolText.Text"=w1719) -> ()  [unwired: 2 in, 2 out]
                      }
                      frame True {
                        n860 = case shown="假" w1730 {
                          tunnel: w1729 -> [_ w1744]
                          tunnel: w1728 -> [w1731 w1745]
                          tunnel: [w1731 w1743] -> w1727
                          tunnel: w1726 -> [_ w1740]
                          tunnel: w1725 -> [_ w1739]
                          tunnel: w1724 -> [_ w1738]
                          tunnel: w1723 -> [_ _]
                          tunnel: w1722 -> [_ w1734]
                          tunnel: w1721 -> [_ w1732]
                          frame False {
                          }
                          frame True {
                            n861 = Quotient & Remainder(x=w1744, y=12) -> (x-y*floor(x/y)=w1736:i32, floor(x/y)=w1735:i32)
                            n862 = Greater Than 0?(x=w1735) -> (x > 0?=w1746:bool)
                            n863 = case shown="真" w1746 {
                              tunnel: w1745 -> [w1762 w1785]
                              tunnel: w1744 -> [_ w1782]
                              tunnel: ["" w1781] -> w1743
                              tunnel: [w1749 w1780] -> w1741
                              tunnel: w1736 -> [w1759 _]
                              tunnel: [w1750 u8 8 ("DataLen")] -> w1737
                              tunnel: w1734 -> [w1748 _]
                              frame False {
                                n864 = Divide(x=w1759, y=2) -> (x/y=w1754:dbl)
                                "发送数据长度" <- w1754
                                n865 = String Subset(string=w1762, length (rest)=w1759) -> (substring=w1752:string)  [unwired: 1 in]
                                n866 = Increment(x=w1754) -> (x+1=w1758:dbl)
                                n867 = Increment(x=w1758) -> (x+1=w1751:dbl)
                                n868 = Quotient & Remainder(x=w1754, y=2.0) -> (x-y*floor(x/y)=w1756:dbl)  [unwired: 1 out]
                                n869 = Equal?(x=w1756, y=1.0) -> (x = y?=w1753:bool)
                                n870 = case shown="真" w1753 {
                                tunnel: w1752 -> [w1763 w1767]
                                tunnel: w1751 -> [w1764 w1769]
                                tunnel: [w1764 w1768] -> w1750
                                tunnel: [w1763 w1766] -> w1749
                                tunnel: w1748 -> [_ w1765]
                                frame False {
                                }
                                frame True {
                                n871 = case shown="\"主板\"" w1765 {
                                tunnel: w1769 -> [w1773 w1776]
                                tunnel: [w1772 w1776] -> w1768
                                tunnel: w1767 -> [w1771 w1775]
                                tunnel: [w1770 w1775] -> w1766
                                frame "主板" {
                                n872 = Concatenate Strings(w1771, "FF") -> (w1770:string)
                                n873 = Increment(x=w1773) -> (x+1=w1772:dbl)
                                }
                                frame "从板", Default {
                                }
                                }
                                }
                                }
                              }
                              frame True {
                                w1779 = 12 ("长度（剩余）")
                                n874 = Subtract(x=w1782, y=12 ("长度（剩余）")) -> (x-y=w1784:i32)
                                n875 = String Subset(string=w1785, offset (0)=w1779, length (rest)=w1784) -> (substring=w1781:string)
                                n876 = String Subset(string=w1785, length (rest)=w1779) -> (substring=w1780:string)  [unwired: 1 in]
                                n877 = local write "发送数据长度"(6.0 ("发送数据长度")) -> ()
                              }
                            }
                            n878 = call "CAN R&W.vi"("设备类型"=w1740, "设备索引"=w1739, "CAN路数"=w1738, "DataLen"=w1737, "写地址/数据"=enum16{"写地址", "写数据"}."写数据", "Data Input"=w1741, "枚举"=w1734, "queue out"=w1732) -> ("发送的数据"=w1733:i32[])  [unwired: 18 in, 1 out]
                            n879 = local write "发送的数据"(w1733) -> ()
                          }
                        }
                      }
                    }
                  }
                }
              }
              frame Enabled {
              }
            }
          }
          frame 251 {
            n880 = disable-structure shown="禁用" {
              disable-tunnel: w1796 -> [w1825 _]
              disable-tunnel: w1795 -> [w1824 _]
              disable-tunnel: w1794 -> [w1823 _]
              disable-tunnel: [w1821 _] -> w1793
              disable-tunnel: w1792 -> [w1820 _]
              disable-tunnel: [w1818 _] -> w1791
              disable-tunnel: w1790 -> [w1817 _]
              disable-tunnel: w1789 -> [w1816 _]
              disable-tunnel: w1788 -> [w1815 _]
              disable-tunnel: w1787 -> [w1807 _]
              disable-tunnel: w1786 -> [w1798 _]
              frame Disabled {
                w1812 = 1 ("索引")
                # "FB"
                n881 = Unbundle(w1798) -> (w1799:u8, w1800:u8, w1801:u8, w1802:u8, w1803:u8, w1804:u8, w1805:u8, w1806:u8)  [unwired: 10 out]
                n882 = Build Array(w1799, w1800, w1801, w1802, w1803, w1804, w1805, w1806) -> (w1797:u8[])
                n883 = local read "发送数据长度"() -> (w1813:dbl)
                n884 = local read "发送的数据"() -> (w1814:i32[])
                n885 = String Length(string=w1820) -> (length=w1822:i32)
                n886 = Array Subset(array=w1814, index=w1812, length=w1813) -> (w1810:i32[])
                n887 = Array Subset(array=w1797, index=w1812, length=w1812) -> (w1809:u8[])
                n888 = Array Size(array=w1817) -> (size(s)=w1819:i32)
                n889 = Greater Than 0?(x=w1822) -> (x > 0?=w1826:bool)
                n890 = Equal?(x=w1810, y=w1809) -> (x = y?=w1811:bool[])
                n891 = And Array Elements(Boolean array=w1811) -> (logical AND=w1808:bool)
                n892 = case shown="真" w1808 {
                  tunnel: w1826 -> [_ w1842]
                  tunnel: w1825 -> [_ w1841]
                  tunnel: w1824 -> [_ w1840]
                  tunnel: w1823 -> [_ w1839]
                  tunnel: w1822 -> [_ w1838]
                  tunnel: [_ w1837] -> w1821
                  tunnel: w1820 -> [_ w1836]
                  tunnel: w1819 -> [_ w1835]
                  tunnel: [_ w1834] -> w1818
                  tunnel: w1817 -> [_ w1833]
                  tunnel: w1816 -> [_ w1832]
                  tunnel: w1815 -> [_ w1831]
                  tunnel: w1807 -> [_ w1830]
                  tunnel: w1807 -> [_ w1829]
                  frame False {
                    w1827 = "失败" ("布尔文本.文本")
                    w1828 = cluster{u32, u32}[] [{16711680, 0}] ("颜色[4]")
                    n893 = property on="烧录结果" class="Bool (严格)"("Colors [4]"=w1828, "BoolText.Text"=w1827) -> ()  [unwired: 2 in, 2 out]
                    n894 = property on="校验" class="Bool (严格)"("Colors [4]"=w1828, "BoolText.Text"=w1827) -> ()  [unwired: 2 in, 2 out]
                  }
                  frame True {
                    n895 = case shown="真" w1842 {
                      tunnel: w1841 -> [w1855 w1955]
                      tunnel: w1840 -> [w1854 w1954]
                      tunnel: w1839 -> [w1853 w1953]
                      tunnel: w1838 -> [_ w1952]
                      tunnel: w1836 -> [_ w1951]
                      tunnel: [w1852 w1950] -> w1837
                      tunnel: w1836 -> [w1851 _]
                      tunnel: w1835 -> [w1848 _]
                      tunnel: w1833 -> [w1856 _]
                      tunnel: [w1850 w1946] -> w1834
                      tunnel: w1833 -> [w1849 w1946]
                      tunnel: w1832 -> [w1845 w1944]
                      tunnel: w1831 -> [w1844 _]
                      tunnel: w1830 -> [_ w1942]
                      tunnel: w1829 -> [w1843 _]
                      frame False {
                        n896 = Greater?(x=w1848, y=0) -> (0:w1846:bool)
                        n897 = case shown="真" w1846 {
                          tunnel: w1856 -> [_ w1904]
                          tunnel: w1855 -> [w1860 w1907]
                          tunnel: w1854 -> [w1859 w1906]
                          tunnel: w1853 -> [w1863 w1905]
                          tunnel: [w1879 w1903] -> w1852
                          tunnel: w1851 -> [w1879 _]
                          tunnel: [w1878 w1902] -> w1850
                          tunnel: w1849 -> [w1878 _]
                          tunnel: w1845 -> [_ w1895]
                          tunnel: w1844 -> [w1865 _]
                          tunnel: w1843 -> [_ w1893]
                          frame False {
                            w1857 = "成功" ("布尔文本.文本")
                            w1858 = cluster{u32, u32}[] [{6618880, 0}] ("颜色[4]")
                            w1873 = u8 0 ("元素")
                            n898 = flat-sequence {
                              tunnel: w1865 -> [w1890]
                              tunnel: [w1890] -> w1864
                              tunnel: [w1892] -> w1866
                              tunnel: w1864 -> [w1892]
                              frame #0 {
                                n899 = invoke on="开始监控 2" class="Bool" method="Reinit To Default"() -> ()  [unwired: 3 in, 3 out]
                                n900 = local write "TEMP"(FALSE ("TEMP")) -> ()
                              }
                              frame #1 {
                                n901 = Wait (ms)(milliseconds to wait=u32 500 ("等待时间（毫秒）")) -> ()  [unwired: 1 out]
                              }
                            }
                            n902 = Bundle(cluster=w1866, "ID"=u32 0, "TimeStamp"=u8 0 ("RemoteFlag"), "TimeFlag"=u8 1, "SendType"=u8 0 ("DataLen"), "RemoteFlag"=u8 0, "ExternFlag"=u8 0, "DataLen"=u8 1, u8 5 ("元素"), w1873, w1873, w1873) -> (w1877:T2)  [unwired: 7 in]
                            n903 = dll-call lib="F:/Bluewave New Energy/SVN_Work/BMS_BootLoader/trunk/BMS_Bootloader/AutoBurn/Settings/ControlCAN.dll" fn="VCI_Transmit"("DeviceType"=w1860, "DeviceInd"=w1859, "CANInd"=w1863, "pSend"=w1877, "Len"=u32 1) -> (error out=w1862:errorcluster)  [unwired: 5 in, 5 out]
                            n904 = local read "Mode"() -> (w1861:bool)
                            n905 = case shown="假" w1861 {
                              tunnel: w1860 -> [_ w1888]
                              tunnel: w1859 -> [_ w1887]
                              tunnel: w1863 -> [_ w1886]
                              tunnel: w1862 -> [_ w1884]
                              frame False {
                                n906 = flat-sequence {
                                frame #0 {
                                n907 = Wait (ms)(milliseconds to wait=u32 500 ("等待时间（毫秒）")) -> ()  [unwired: 1 out]
                                }
                                frame #1 {
                                n908 = local write "TEMP"(TRUE ("TEMP")) -> ()
                                n909 = local write "连接状态"(TRUE ("CAN连接状态")) -> ()
                                }
                                }
                              }
                              frame True {
                                n910 = invoke on="开始监控" class="Bool" method="Reinit To Default"() -> ()  [unwired: 3 in, 3 out]
                                n911 = local write "连接状态"(FALSE ("CAN连接状态")) -> ()
                                n912 = call "CAN_Init.vi"("设备类型"=w1888, "设备索引"=w1887, "CAN路数"=w1886, "操作类型"=enum16{"初始化CAN", "关闭CAN"}."关闭CAN", "error in (no error)"=w1884) -> ()  [unwired: 13 in, 2 out]
                              }
                            }
                            n913 = property on="烧录结果" class="Bool (严格)"("Colors [4]"=w1858, "BoolText.Text"=w1857) -> ()  [unwired: 2 in, 2 out]
                            n914 = invoke on="Monitor" class="Bool" method="Reinit To Default"() -> ()  [unwired: 3 in, 3 out]
                            n915 = property on="校验" class="Bool (严格)"("Colors [4]"=w1858, "BoolText.Text"=w1857) -> ()  [unwired: 2 in, 2 out]
                          }
                          frame True {
                            w1897 = 100.0 ("y")
                            n916 = Delete From Array(array=w1904, length=1 ("长度"), index=0 ("索引")) -> (array with subset deleted=w1902:string[])  [unwired: 1 out]
                            n917 = local read "大小"() -> (w1900:i32)
                            n918 = Array Size(array=w1902) -> (size(s)=w1901:i32)
                            n919 = Index Array(array=w1904, index=0 ("索引")) -> (element=w1912:string)
                            n920 = Divide(x=w1901, y=w1900) -> (x/y=w1899:dbl)
                            n921 = String Subset(string=w1912, offset (0)=0 ("偏移量(0)"), length (rest)=2 ("长度（剩余）")) -> (substring=w1919:string)
                            n922 = String Subset(string=w1912, offset (0)=2 ("偏移量(0)"), length (rest)=2 ("长度（剩余）")) -> (substring=w1922:string)
                            n923 = Multiply(x=w1899, y=w1897) -> (x*y=w1898:dbl)
                            n924 = Subtract(x=w1897, y=w1898) -> (x-y=w1896:dbl)
                            n925 = Hexadecimal String To Number(string=w1922) -> (number=w1917:u32)  [unwired: 2 in, 1 out]
                            n926 = case shown="\"S1\", 默认" w1919 {
                              tunnel: [4 ("偏移量(0)") 6 ("偏移量(0)")] -> w1911
                              tunnel: w1917 -> [w1934 w1940]
                              tunnel: [w1932 w1938] -> w1916
                              tunnel: [8 ("y") 10 ("y")] -> w1913
                              tunnel: ["S1" "S2"] -> w1908
                              frame "S1", Default {
                                n927 = Subtract(x=w1934, y=3) -> (x-y=w1932:u32)
                              }
                              frame "S2" {
                                n928 = Subtract(x=w1940, y=4) -> (x-y=w1938:u32)
                              }
                            }
                            "地址长度 2" <- w1911
                            n929 = local write "进度"(w1896) -> ()
                            n930 = String Subset(string=w1912, offset (0)=4 ("偏移量(0)"), length (rest)=w1911) -> ()  [unwired: 1 out]
                            n931 = Multiply(x=u32 2, y=w1916) -> (x*y=w1914:u32)
                            "数据长度 2" <- w1914
                            n932 = String Subset(string=w1912, offset (0)=4 ("偏移量(0)"), length (rest)=w1911) -> (substring=w1909:string)
                            n933 = call "CAN R&W.vi"("设备类型"=w1907, "设备索引"=w1906, "CAN路数"=w1905, "DataLen"=u8 8, "写地址/数据"=enum16{"写地址", "写数据"}."写地址", "Data Input"=w1909, "枚举"=w1895, "TYPE"=w1908, "queue out"=w1893) -> ("发送的数据"=w1894:i32[])  [unwired: 17 in, 1 out]
                            n934 = local write "发送的数据"(w1894) -> ()
                            n935 = String Subset(string=w1912, offset (0)=w1913, length (rest)=w1914) -> (substring=w1903:string)
                            "子字符串 2" <- w1903
                          }
                        }
                      }
                      frame True {
                        n936 = Quotient & Remainder(x=w1952, y=12) -> (x-y*floor(x/y)=w1947:i32, floor(x/y)=w1948:i32)
                        n937 = Greater Than 0?(x=w1948) -> (x > 0?=w1957:bool)
                        n938 = case shown="假" w1957 {
                          tunnel: w1951 -> [w1977 w2002]
                          tunnel: w1952 -> [_ w1999]
                          tunnel: ["" w1998] -> w1950
                          tunnel: [w1962 w1997] -> w1945
                          tunnel: w1947 -> [w1975 _]
                          tunnel: [w1963 u8 8 ("DataLen")] -> w1949
                          tunnel: w1946 -> [w1972 _]
                          tunnel: w1944 -> [w1961 _]
                          frame False {
                            n939 = Divide(x=w1975, y=2) -> (x/y=w1960:dbl)
                            n940 = Array Size(array=w1972) -> (size(s)=w1971:i32)
                            n941 = String Subset(string=w1977, length (rest)=w1975) -> (substring=w1965:string)  [unwired: 1 in]
                            n942 = Increment(x=w1960) -> (x+1=w1973:dbl)
                            n943 = Increment(x=w1973) -> (x+1=w1964:dbl)
                            n944 = Equal?(x=0, y=w1971) -> (x = y?=w1959:bool)
                            n945 = Quotient & Remainder(x=w1960, y=2.0) -> (x-y*floor(x/y)=w1968:dbl)  [unwired: 1 out]
                            n946 = local write "发送数据长度"(w1960) -> ()
                            n947 = Equal?(x=w1968, y=1.0) -> (x = y?=w1966:bool)
                            n948 = case shown="真" w1959 {
                              frame False {
                              }
                              frame True {
                                w1978 = "成功" ("布尔文本.文本")
                                w1979 = cluster{u32, u32}[] [{6618880, 0}] ("颜色[4]")
                                n949 = invoke on="Monitor" class="Bool" method="Reinit To Default"() -> ()  [unwired: 3 in, 3 out]
                                n950 = property on="烧录结果" class="Bool (严格)"("Colors [4]"=w1979, "BoolText.Text"=w1978) -> ()  [unwired: 2 in, 2 out]
                                n951 = property on="校验" class="Bool (严格)"("Colors [4]"=w1979, "BoolText.Text"=w1978) -> ()  [unwired: 2 in, 2 out]
                              }
                            }
                            n952 = case shown="假" w1966 {
                              tunnel: w1965 -> [w1980 w1984]
                              tunnel: w1964 -> [w1981 w1986]
                              tunnel: [w1981 w1985] -> w1963
                              tunnel: [w1980 w1983] -> w1962
                              tunnel: w1961 -> [_ w1982]
                              frame False {
                              }
                              frame True {
                                n953 = case shown="\"主板\"" w1982 {
                                tunnel: w1986 -> [w1991 w1993]
                                tunnel: [w1990 w1993] -> w1985
                                tunnel: w1984 -> [w1989 w1992]
                                tunnel: [w1987 w1992] -> w1983
                                frame "主板" {
                                n954 = Concatenate Strings(w1989, "FF") -> (w1987:string)
                                n955 = Increment(x=w1991) -> (x+1=w1990:dbl)
                                }
                                frame "从板", Default {
                                }
                                }
                              }
                            }
                          }
                          frame True {
                            w1996 = 12 ("长度（剩余）")
                            n956 = Subtract(x=w1999, y=12 ("长度（剩余）")) -> (x-y=w2001:i32)
                            n957 = String Subset(string=w2002, offset (0)=w1996, length (rest)=w2001) -> (substring=w1998:string)
                            n958 = String Subset(string=w2002, length (rest)=w1996) -> (substring=w1997:string)  [unwired: 1 in]
                            n959 = local write "发送数据长度"(6.0 ("发送数据长度")) -> ()
                          }
                        }
                        n960 = call "CAN R&W.vi"("设备类型"=w1955, "设备索引"=w1954, "CAN路数"=w1953, "DataLen"=w1949, "写地址/数据"=enum16{"写地址", "写数据"}."写数据", "Data Input"=w1945, "枚举"=w1944, "queue out"=w1942) -> ("发送的数据"=w1943:i32[])  [unwired: 18 in, 1 out]
                        n961 = local write "发送的数据"(w1943) -> ()
                      }
                    }
                  }
                }
              }
              frame Enabled {
              }
            }
          }
          frame 1, Default {
            (unwired) TRUE
            # "040000"
            n962 = local read "请选择板号"() -> (w2007:u16)
            n963 = Increment(x=w2007) -> (x+1=w2006:u16)
            n964 = Subtract(x=w2008, y=w2006) -> (x-y=w2005:u32)
            n965 = case shown="4010000" w2005 {
              tunnel: w2004 -> [_ w2011 w2016]
              tunnel: w2003 -> [_ _ w2015]
              frame 0, Default {
              }
              frame 67108864 {
                n966 = local write "Life"(w2011) -> ()
              }
              frame 67174400 {
                n967 = Join Numbers(hi=w2016, lo=w2015) -> ((hi.lo)=w2014:u16)
                n968 = Divide(x=w2014, y=u16 10) -> (x/y=→"总电压":dbl)
              }
            }
          }
        }
      }
    }
  }
  n969 = property on="手动进入编程模式" class="Bool (严格)"("DisabledEnum"=T3."Disabled and Grayed Out" ("禁用")) -> ()  [unwired: 2 in, 2 out]
  n970 = local write "开始下载数据"(FALSE ("开始下载数据")) -> ()
  n971 = Release Queue(queue=w3, error in (no error)=w2) -> ()  [unwired: 1 in, 3 out]
  n972 = local write "start"(u32 0 ("start")) -> ()
  n973 = Build Array(cluster{u32, u32} {0, 0}) -> (w27:cluster{u32, u32}[])
  n974 = local write "Info："("" ("字符串")) -> ()
  n975 = local write "进入烧录"(FALSE ("进入烧录")) -> ()
  n976 = property on="MD5校验" class="Bool (严格)"("Colors [4]"=w27, "BoolText.Text"="失败" ("布尔文本.文本")) -> ()  [unwired: 2 in, 2 out]
  n977 = local write "子数组"(string[] ["  "] ("子数组")) -> ()
  n978 = local write "发送数据长度"(0.0 ("发送数据长度")) -> ()
  n979 = local write "擦除完成"(w37) -> ()
  n980 = local write "进入烧录模式"(w37) -> ()
  "连接状态" <- FALSE ("CAN连接状态")
  "CAN数据" <- FALSE ("烧录中")
  "进度" <- u8 0 ("进度")
  "烧录结果" <- FALSE ("烧录完成")
  "Mode" <- TRUE ("Mode")
  "update flag" <- FALSE
